vi "HighLVL.vi"() -> ()   [LabVIEW 2015]
uses:
  Public/Documents/SItoolkit/LabVIEW/Examples2015_6_0_2_9/Fast Examples/Open-Close Hardware/CamHandle.vi
  Public/Documents/SItoolkit/LabVIEW/Examples2015_6_0_2_9/Fast Examples/Cameras/NumericIndicator.vi
panel:
  out "Boolean":bool
  out "?":dbl
  out "Progress":u8(slide) scale=0.0..100.0
  out "Source Voltage":dbl
  out "Current (mA)":dbl
  out "Diode 2":string
  out "Diode 1":string
  out "Diode 3":string
  in  "File Path for Data Log":path=path "C:/Users/user/Dropbox (MIT)/stats/stats_00_00_00.txt"
  out "Source Mirror Position (mm)":dbl(slide) scale=0.0..50.0 scale format="%#.6g"
  out "Camera\nClosed":bool
  out "error out (Shutoff)":errorcluster
  out "Experiment Complete":bool
  out "Current File":string
  out "Logging Indicator":bool
  out "Current Set":dbl
  out "Current Frame":dbl
  in  "Anode":i32(knob) scale=1.0..6.0
  in  "Base FilePath (incrementing counter will be added to each following dataset)":path=path "C:/Users/Polarimetry/Desktop/High level experiment/exp"
  in  "Axis Positions":T1
  out "Experiment \nStarted":bool
  out "Estimated time (min)":dbl
  out "Initializing":bool
  out "error out (ADC)":errorcluster
  in  "begin":bool
  out "Read Temp":dbl(slide) scale=-50.0..20.0
  out "Camera open":bool
  out "Y Dimension":u32
  out "X Dimension":u32
  out "error out (Open Cam)":errorcluster
  in  "error in (no error)":errorcluster
  in  "Experiment Parameters":T2(tab)
  in  "Throwaway Frames":i32=1
  in  "# Frames":i32=10
  in  "ADC Speed (kHz)":i32=100
  in  "Exposure":i32=45
  in  "Cooling Temp":dbl=-50.0
  in  "Y2":i32=1300
  in  "Y1":i32=1
  in  "X2":i32=1340
  in  "X1":i32=1
  in  "x bin":u32=1
  in  "y bin":u32=1
  in  "min block":u32=2
  in  "Num Min Block":u32=5
  in  "ADC port":i32=1
  in  "ADC gain":i32=-1
  in  "Timing Mode":u32(ring)=1 items=["N/A", "Timed Mode/Free run", "Trigger First (only PM)", "Strobed/Ext Sync", "Bulb Mode (PM only)", "Variable Timed mode (PM only)", "Flash Mode (only some PM)"]
  in  "Motor Controls":T3(tab)
  in  "Detector Y#Steps":i32=1
  in  "Detector Y End":dbl
  in  "Detector Y Start":dbl
  in  "Detector X#Steps":i32=1
  in  "Detector X End":dbl
  in  "Detector X Start":dbl
  in  "Grating Angle#Steps":i32=1
  in  "Grating Angle End":dbl
  in  "Grating Angle Start":dbl
  in  "Grating Y#Steps":i32=1
  in  "Grating Y End":dbl
  in  "Grating Y Start":dbl
  in  "Grating X#Steps":i32=1
  in  "Grating X End":dbl
  in  "Grating X Start":dbl
  in  "Aperture X#Steps":i32=1
  in  "Aperture X End":dbl
  in  "Aperture X Start":dbl
  in  "Polarization #Steps":i32=1
  in  "Polarization End":dbl
  in  "Polarization Start":dbl
  in  "Mirror Angle #Steps":i32=1
  in  "Mirror Angle End":dbl
  in  "Mirror Angle Start":dbl
  in  "Mirror X #Steps":i32=1
  in  "Mirror X End":dbl
  in  "Mirror X Start":dbl
  # "These should be 1340 and 1300,\n if not, it is a demo cam"
  # "Note: Anode motor is not set up. \nOnly change this here if you manually changed the anode"
  # "Logging"
  # "ROI"
  # "Anode Control Not Supported.\nShut Off Voltage and Try Manually."
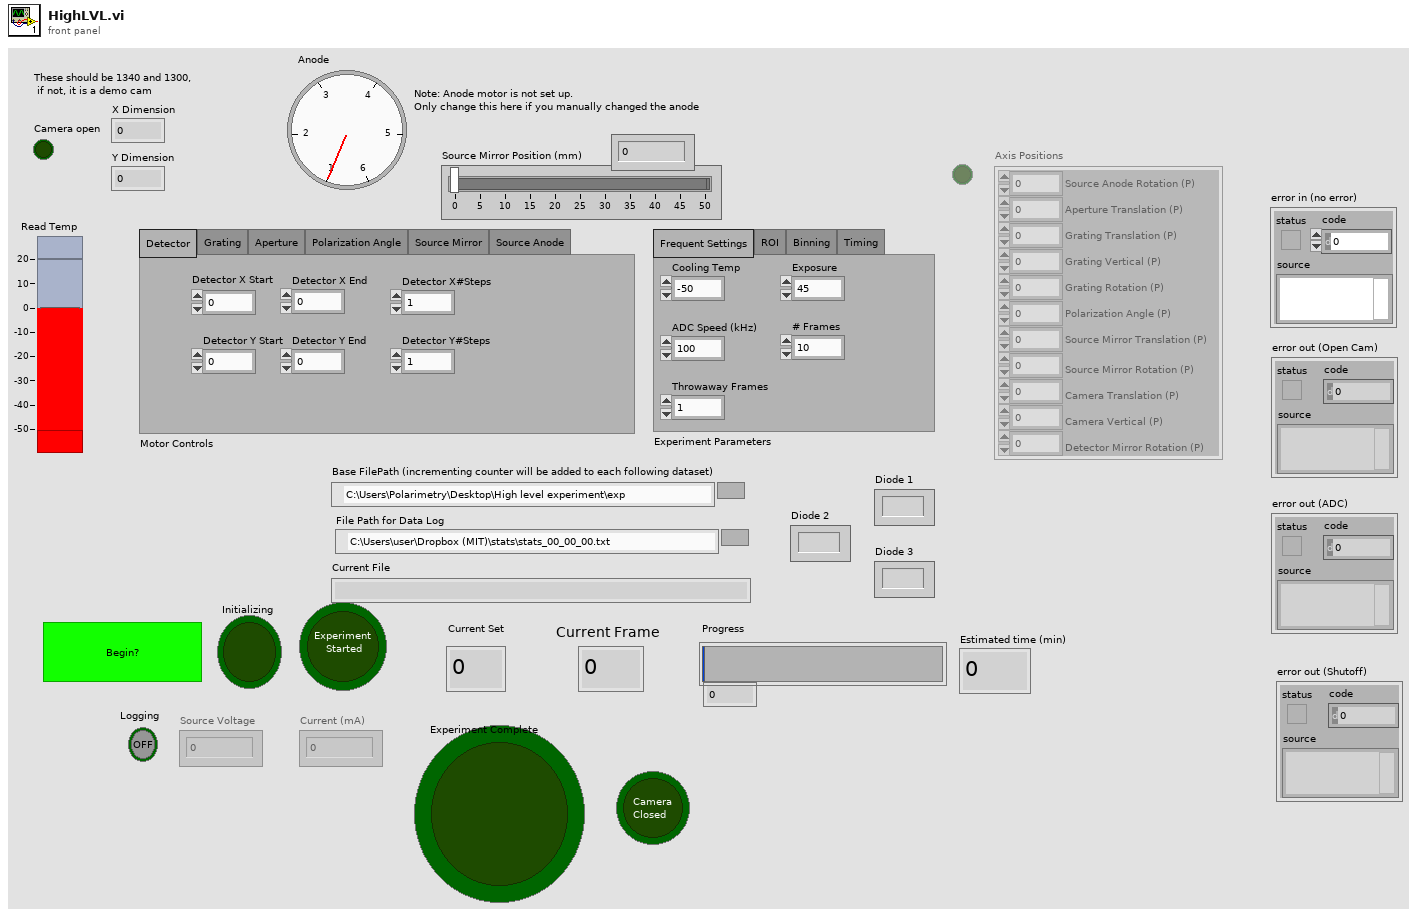
[diagram p1: front panel]
types:
  T1 = cluster{"Source Anode Rotation (P)":dbl, "Aperture Translation (P)":dbl, "Grating Translation (P)":dbl, "Grating Vertical (P)":dbl, "Grating Rotation (P)":dbl, "Polarization Angle (P)":dbl, "Source Mirror Translation (P)":dbl, "Source Mirror Rotation (P)":dbl, "Camera Translation (P)":dbl, "Camera Vertical (P) ":dbl, "Detector Mirror Rotation (P)":dbl}
  T2 = enum32{"Frequent Settings", "ROI", "Binning", "Timing"}
  T3 = enum32{"Detector", "Grating", "Aperture", "Polarization Angle", "Source Mirror", "Source Anode"}
  T4 = cluster{"Axis Prefix":string, bool, i32, i32, i32, i32}
  T5 = cluster{"Axis Prefix":string, bool, i32, i32, i32, dbl}
  T6 = cluster{"Axis Prefix":string, bool, i32, dbl, i32, i32}
  T7 = enum16{"open", "replace", "create", "open or create", "replace or create", "replace or create with confirmation"}
  T8 = cluster{"Detector X Start":dbl, "Detector Y Start":dbl, "Grating X Start":dbl, "Grating Y Start":dbl, "Grating Angle Start":dbl, "Aperture X Start":dbl, "Polarization Start":dbl, "Mirror X Start":dbl, "Mirror Angle Start":dbl}
  T9 = cluster{"Detector X End":dbl, "Detector Y End":dbl, "Grating X End":dbl, "Grating Y End":dbl, "Grating Angle End":dbl, "Aperture X End":dbl, "Polarization End":dbl, "Mirror X End":dbl, "Mirror Angle End":dbl}
  T10 = cluster{"Detector X#Steps":i32, "Detector Y#Steps":i32, "Grating X#Steps":i32, "Grating Y#Steps":i32, "Grating Angle#Steps":i32, "Aperture X#Steps":i32, "Polarization #Steps":i32, "Mirror X #Steps":i32, "Mirror Angle #Steps":i32}
  T11 = cluster{"ADC Speed (kHz)":i32, "Throwaway Frames":i32, "# Frames":i32, "Exposure":i32, "Cooling Temp":dbl}
  T12 = cluster{"X1":i32, "X2":i32, "x bin":u32, "Y1":i32, "Y2":i32, "y bin":u32}
  T13 = cluster{"Increment":dbl, "Increment":dbl, "Increment":dbl, "Increment":dbl, "Increment":dbl, "Increment":dbl, "Increment":dbl, "Increment":dbl, "Increment":dbl}
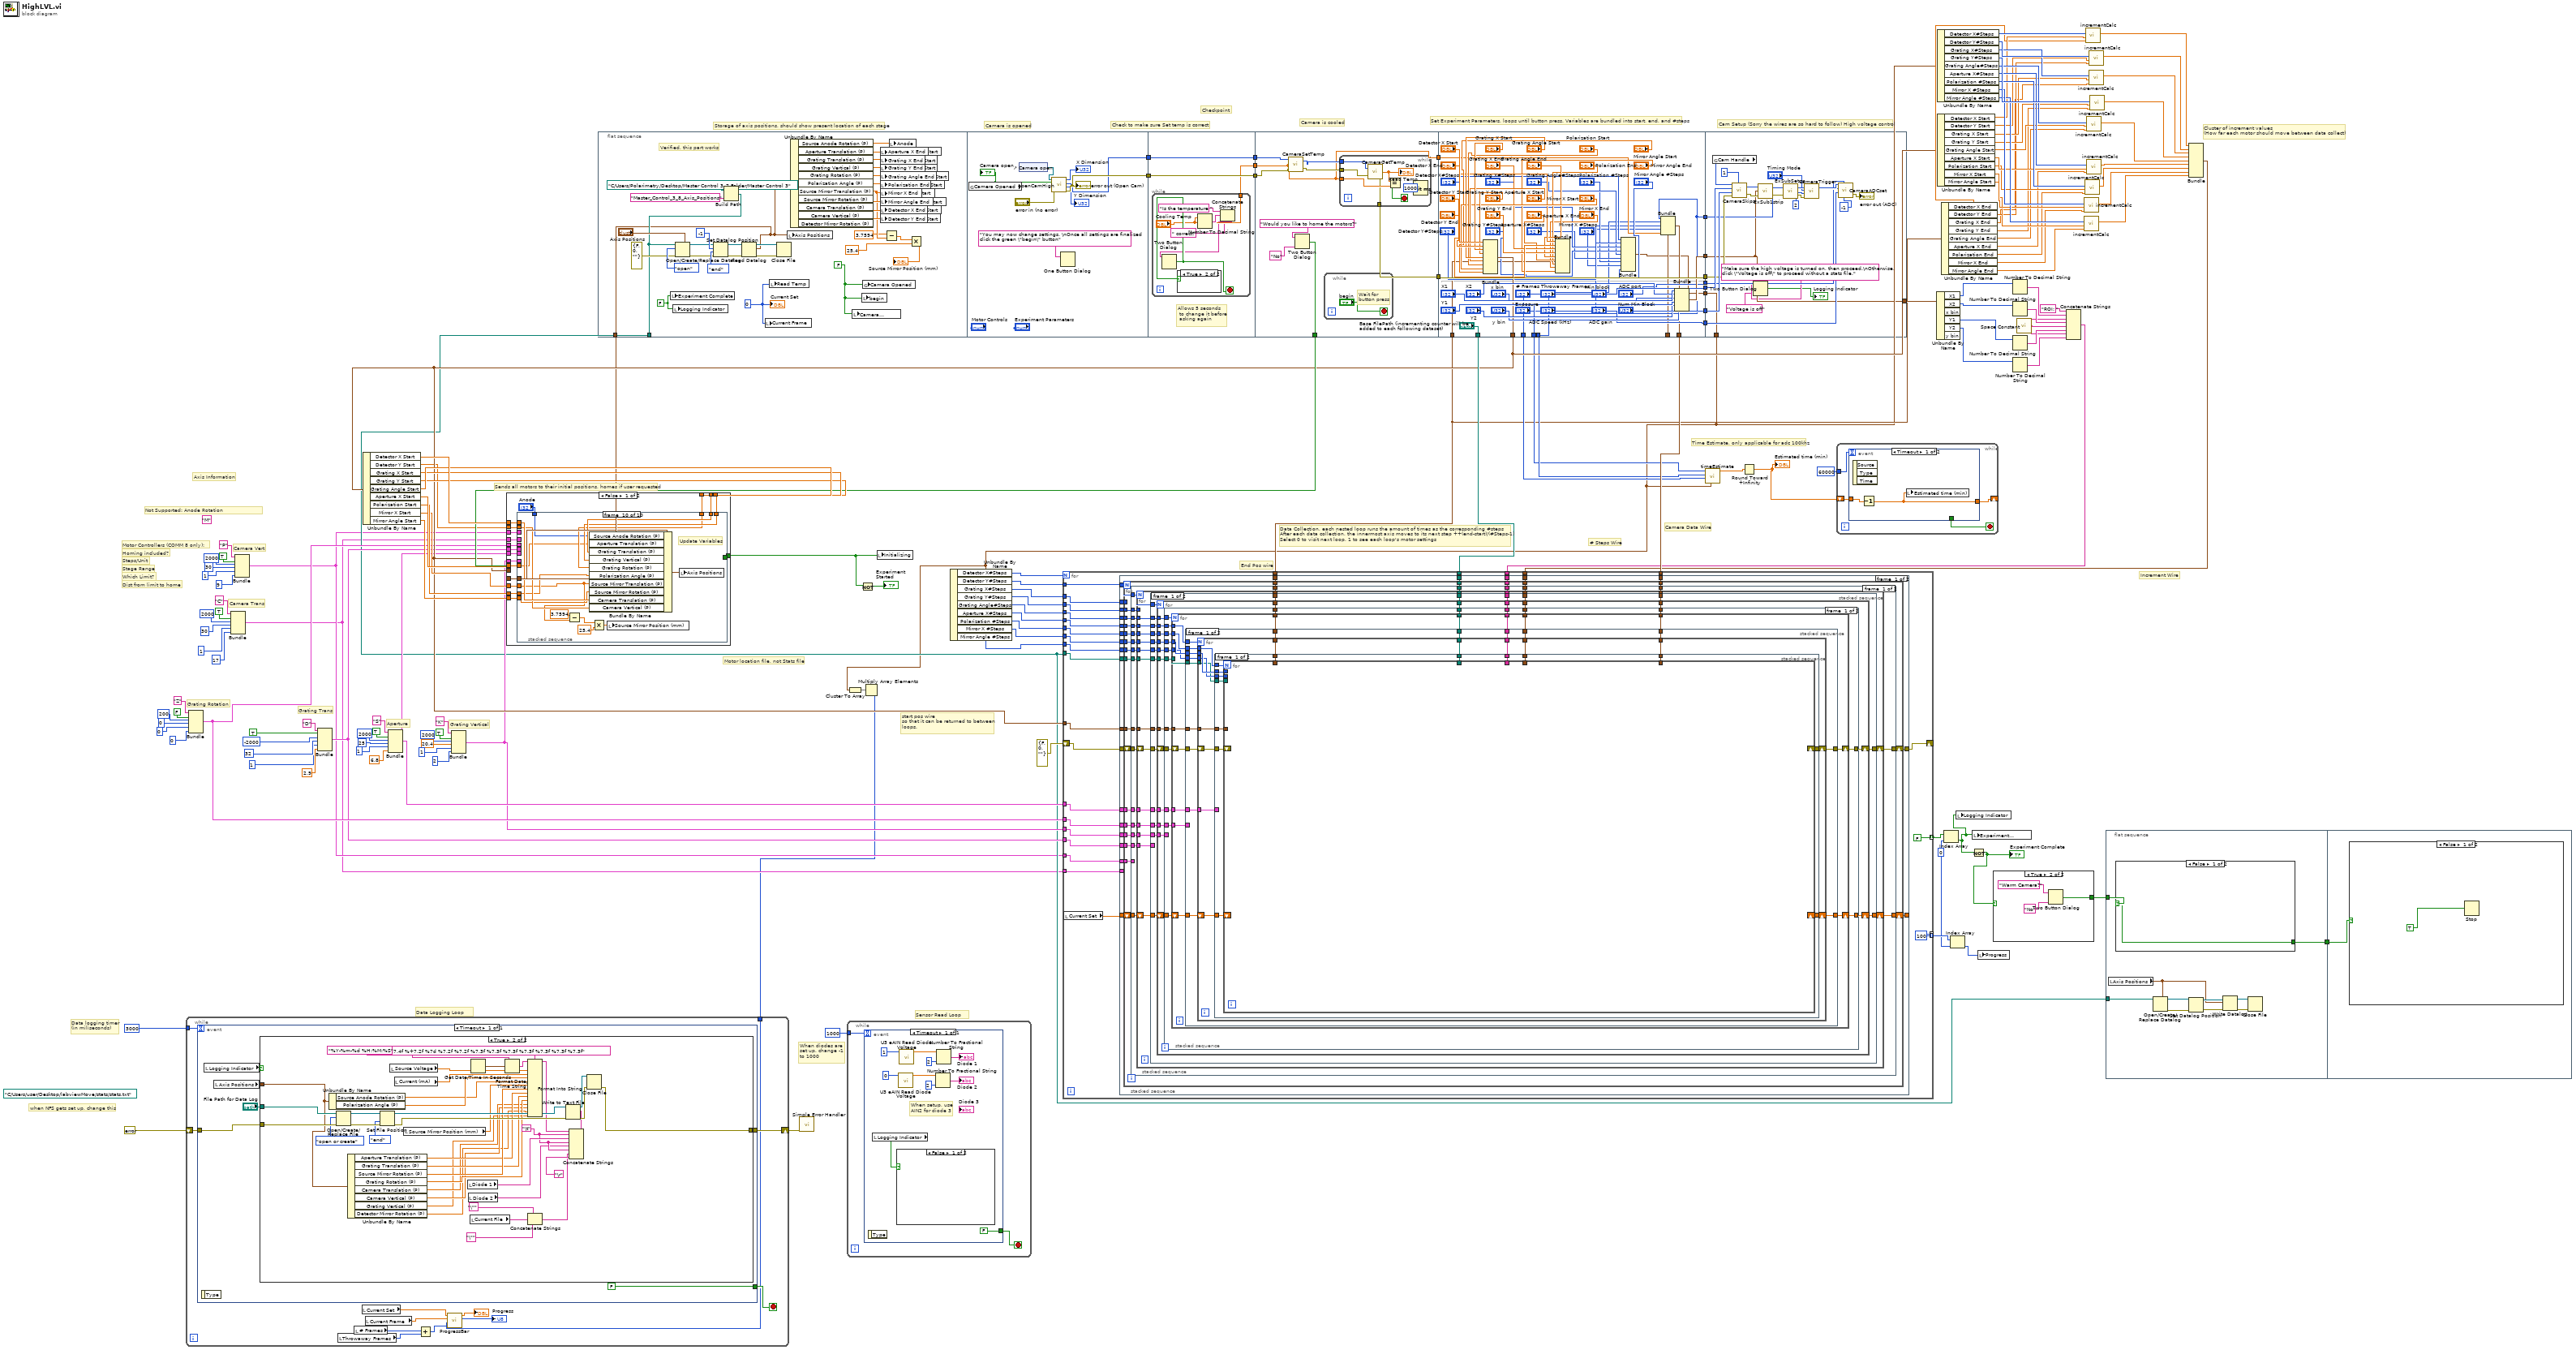
[diagram p0: block diagram]
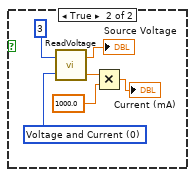
[diagram p2: hidden frame]
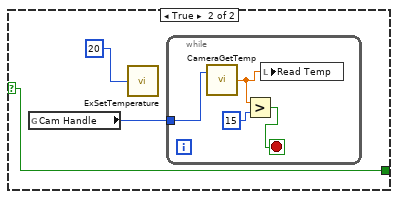
[diagram p4: hidden frame]
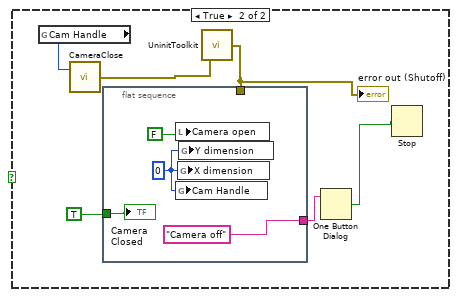
[diagram p5: hidden frame]
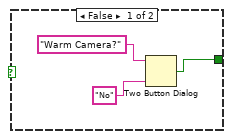
[diagram p6: hidden frame]
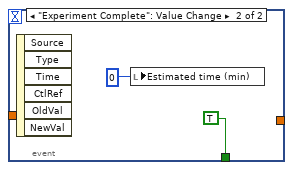
[diagram p7: hidden frame]
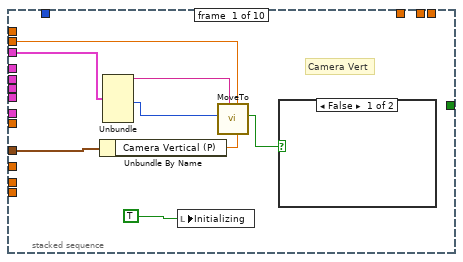
[diagram p8: hidden frame]
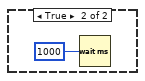
[diagram p9: hidden frame]
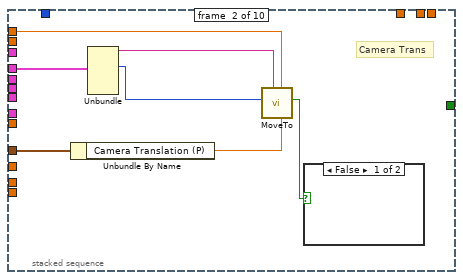
[diagram p10: hidden frame]
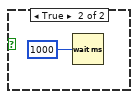
[diagram p11: hidden frame]
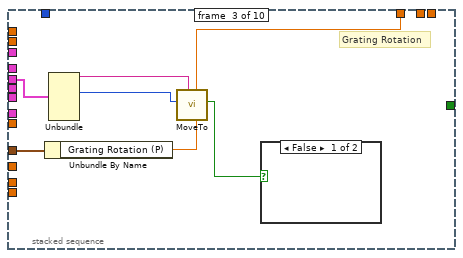
[diagram p12: hidden frame]
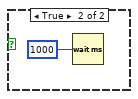
[diagram p13: hidden frame]
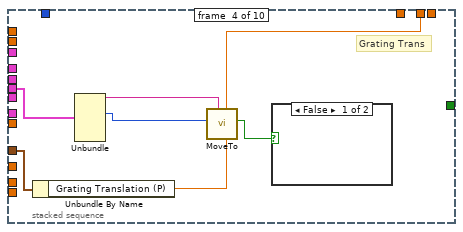
[diagram p14: hidden frame]
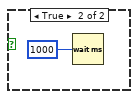
[diagram p15: hidden frame]
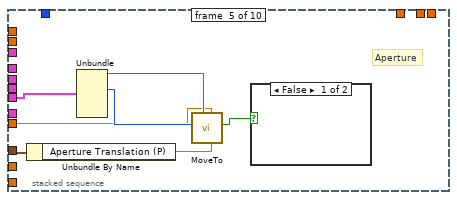
[diagram p16: hidden frame]
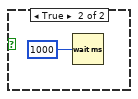
[diagram p17: hidden frame]
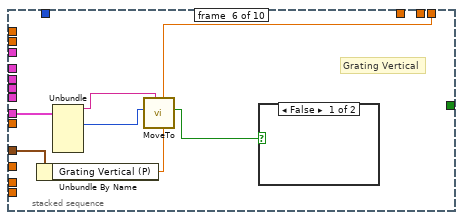
[diagram p18: hidden frame]
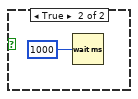
[diagram p19: hidden frame]
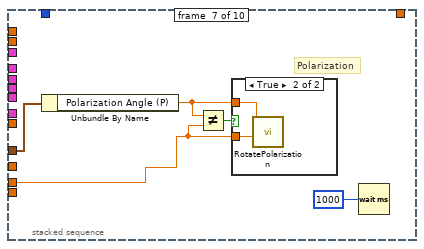
[diagram p20: hidden frame]
diagram:
  (unwired) path "C:/Users/user/Desktop/labviewMove/stats/stats.txt" ("file path (use dialog)")
  w3 = 0
  (unwired) "M" ("Axis Prefix")
  # "when NFS gets set up, change this"
  # "When diodes are \nset up, change -1 \nto 1000"
  # "Sensor Read Loop"
  # "Data Logging Loop"
  # "Data logging timer\n(in miliseconds)"
  # "Checkpoint"
  # "Motor location file, not Stats file"
  # "Increment Wire"
  # "Camera Data Wire"
  # "# Steps Wire"
  # "End Pos wire"
  # "start pos wire\nso that it can be returned to between\nloops."
  # "Cluster of increment values \n(How far each motor should move between data collect)"
  # "Storage of axis positions, should show present location of each stage"
  # "Data Collection, each nested loop runs the amount of times as the corresponding #steps\nAfter each data collection, the innermost axis moves to its next step ++(end-start)/(#Steps-1)\nSelect 0 to visit next loop, 1 to see each loop's motor settings"
  # "Time Estimate, only applicable for adc 100khz"
  # "Axis Information"
  # "Camera Vert"
  # "Camera Trans"
  # "Grating Rotation"
  # "Grating Vertical"
  # "Grating Trans"
  # "Aperture"
  # "Dist from limit to home"
  # "Not Supported: Anode Rotation"
  # "Which Limit?"
  # "Stage Range"
  # "Steps/Unit"
  # "Homing included?"
  # "Motor Controllers (COMM 8 only):"
  # "Sends all motors to their initial positions, homes if user requested"
  # "Cam Setup (Sorry the wires are so hard to follow) High voltage control"
  # "Check to make sure Set temp is correct"
  # "Set Experiment Parameters, loops until button press. Variables are bundled into start, end, and #steps"
  # "Camera is cooled"
  # "Camera is opened"
  n1 = Bundle("Axis Prefix"="Z", FALSE, 200, 0, 0, 0) -> (w29:T4)  [unwired: 1 in]
  n2 = Bundle("Axis Prefix"="C", TRUE, 2000, 30, 1, 17) -> (w11:T4)  [unwired: 1 in]
  n3 = Bundle("Axis Prefix"="P", TRUE, 2000, 30, 1, 9) -> (w12:T4)  [unwired: 1 in]
  n4 = Bundle("Axis Prefix"="D", TRUE, -2000, 32, 1, 2.9) -> (w22:T5)  [unwired: 1 in]
  n5 = Unbundle By Name(w50) -> ("Detector X Start"=w145:dbl, "Detector Y Start"=w23:dbl, "Grating X Start"=w107:dbl, "Grating Y Start"=w105:dbl, "Grating Angle Start"=w108:dbl, "Aperture X Start"=w106:dbl, "Polarization Start"=w90:dbl, "Mirror X Start"=w89:dbl, "Mirror Angle Start"=w88:dbl)
  n6 = Bundle("Axis Prefix"="S", TRUE, 2000, 25, 1, 6.8) -> (w30:T5)  [unwired: 1 in]
  n7 = Bundle("Axis Prefix"="K", TRUE, 2000, 20.4, 1, 2) -> (w28:T6)  [unwired: 1 in]
  n8 = case shown="False" w51 {
    tunnel: w145 -> [w173 w279]
    tunnel: w12 -> [w172 w278]
    tunnel: w11 -> [w168 w277]
    tunnel: w29 -> [w169 w276]
    tunnel: w22 -> [w166 w275]
    tunnel: w30 -> [w164 w274]
    tunnel: w28 -> [w162 w273]
    tunnel: w23 -> [w170 w272]
    tunnel: w108 -> [w167 w271]
    tunnel: w107 -> [w165 w270]
    tunnel: w106 -> [w163 w269]
    tunnel: w105 -> [w161 w268]
    tunnel: [w157 w267] -> w95
    tunnel: w21 -> [w171 w266]
    tunnel: w90 -> [w159 w265]
    tunnel: w89 -> [w160 w264]
    tunnel: w88 -> [w158 w263]
    tunnel: w50 -> [_ w262]
    frame False {
      n9 = stacked-sequence {
        tunnel: w173 -> [_ w183 _ _ _ _ _ _ _ w259]
        tunnel: w172 -> [w181 _ _ _ _ _ _ _ _ _]
        tunnel: w171 -> [w178 w187 w195 w201 w213 w218 w227 w233 w241 w260]
        tunnel: w170 -> [w174 _ _ _ _ _ _ _ _ w258]
        tunnel: w169 -> [_ _ w191 _ _ _ _ _ _ _]
        tunnel: w168 -> [_ w185 _ _ _ _ _ _ _ _]
        tunnel: w167 -> [_ _ w193 _ _ _ _ _ _ w255]
        tunnel: w166 -> [_ _ _ w205 _ _ _ _ _ _]
        tunnel: w165 -> [_ _ _ w202 _ _ _ _ _ w257]
        tunnel: w164 -> [_ _ _ _ w211 _ _ _ _ _]
        tunnel: w163 -> [_ _ _ _ w207 _ _ _ _ w253]
        tunnel: w162 -> [_ _ _ _ _ w221 _ _ _ _]
        tunnel: w161 -> [_ _ _ _ _ w216 _ _ _ w256]
        tunnel: "Anode" -> [_ _ _ _ _ _ _ _ _ w254]
        tunnel: w160 -> [_ _ _ _ _ _ _ w231 _ w246]
        tunnel: w159 -> [_ _ _ _ _ _ w224 _ _ w252]
        tunnel: w158 -> [_ _ _ _ _ _ _ _ w237 w251]
        tunnel: [_ _ _ _ _ _ _ _ FALSE _] -> w157
        frame #0 {
          # "Camera Vert"
          n10 = Unbundle By Name(w178) -> ("Camera Vertical (P)"=w177:dbl)
          n11 = Unbundle(w181) -> ("Axis Prefix"=w180:string, w179:i32)  [unwired: 4 out]
          n12 = local write "Initializing"(TRUE) -> ()
          n13 = call "MoveTo.vi"("Curr Pos"=w177, "Desired Pos"=w174, "Axis Name"=w180, "Steps/unit"=w179) -> ("Anything move?"=w176:bool)  [unwired: 7 in]
          n14 = case shown="False" w176 {
            frame False {
            }
            frame True {
              n15 = Wait (ms)(milliseconds to wait=1000) -> ()  [unwired: 1 out]
            }
          }
        }
        frame #1 {
          # "Camera Trans"
          n16 = Unbundle By Name(w187) -> ("Camera Translation (P)"=w186:dbl)
          n17 = Unbundle(w185) -> ("Axis Prefix"=w189:string, w188:i32)  [unwired: 4 out]
          n18 = call "MoveTo.vi"("Curr Pos"=w186, "Desired Pos"=w183, "Axis Name"=w189, "Steps/unit"=w188) -> ("Anything move?"=w184:bool)  [unwired: 7 in]
          n19 = case shown="False" w184 {
            frame False {
            }
            frame True {
              n20 = Wait (ms)(milliseconds to wait=1000) -> ()  [unwired: 1 out]
            }
          }
        }
        frame #2 {
          # "Grating Rotation"
          n21 = Unbundle By Name(w195) -> ("Grating Rotation (P)"=w194:dbl)
          n22 = Unbundle(w191) -> ("Axis Prefix"=w197:string, w196:i32)  [unwired: 4 out]
          n23 = call "MoveTo.vi"("Curr Pos"=w194, "Desired Pos"=w193, "Axis Name"=w197, "Steps/unit"=w196) -> ("Anything move?"=w192:bool)  [unwired: 7 in]
          n24 = case shown="False" w192 {
            frame False {
            }
            frame True {
              n25 = Wait (ms)(milliseconds to wait=1000) -> ()  [unwired: 1 out]
            }
          }
        }
        frame #3 {
          # "Grating Trans"
          n26 = Unbundle By Name(w201) -> ("Grating Translation (P)"=w200:dbl)
          n27 = Unbundle(w205) -> ("Axis Prefix"=w204:string, w203:i32)  [unwired: 4 out]
          n28 = call "MoveTo.vi"("Curr Pos"=w200, "Desired Pos"=w202, "Axis Name"=w204, "Steps/unit"=w203) -> ("Anything move?"=w199:bool)  [unwired: 7 in]
          n29 = case shown="False" w199 {
            frame False {
            }
            frame True {
              n30 = Wait (ms)(milliseconds to wait=1000) -> ()  [unwired: 1 out]
            }
          }
        }
        frame #4 {
          # "Aperture"
          n31 = Unbundle By Name(w213) -> ("Aperture Translation (P)"=w212:dbl)
          n32 = Unbundle(w211) -> ("Axis Prefix"=w210:string, w209:i32)  [unwired: 4 out]
          n33 = call "MoveTo.vi"("Curr Pos"=w212, "Desired Pos"=w207, "Axis Name"=w210, "Steps/unit"=w209) -> ("Anything move?"=w208:bool)  [unwired: 7 in]
          n34 = case shown="False" w208 {
            frame False {
            }
            frame True {
              n35 = Wait (ms)(milliseconds to wait=1000) -> ()  [unwired: 1 out]
            }
          }
        }
        frame #5 {
          # "Grating Vertical"
          n36 = Unbundle By Name(w218) -> ("Grating Vertical (P)"=w217:dbl)
          n37 = Unbundle(w221) -> ("Axis Prefix"=w220:string, w219:i32)  [unwired: 4 out]
          n38 = call "MoveTo.vi"("Curr Pos"=w217, "Desired Pos"=w216, "Axis Name"=w220, "Steps/unit"=w219) -> ("Anything move?"=w215:bool)  [unwired: 7 in]
          n39 = case shown="False" w215 {
            frame False {
            }
            frame True {
              n40 = Wait (ms)(milliseconds to wait=1000) -> ()  [unwired: 1 out]
            }
          }
        }
        frame #6 {
          # "Polarization"
          n41 = Unbundle By Name(w227) -> ("Polarization Angle (P)"=w225:dbl)
          n42 = Not Equal?(x=w225, y=w224) -> (x != y?=w223:bool)
          n43 = case shown="True" w223 {
            tunnel: w224 -> [_ w229]
            tunnel: w225 -> [_ w228]
            frame False {
            }
            frame True {
              n44 = call "RotatePolarization.vi"("End Pos"=w229, "curr pos"=w228) -> ()  [unwired: 9 in, 1 out]
            }
          }
          n45 = Wait (ms)(milliseconds to wait=1000) -> ()  [unwired: 1 out]
        }
        frame #7 {
          # "Mirror X"
          n46 = Unbundle By Name(w233) -> ("Source Mirror Translation (P)"=w230:dbl)
          n47 = Not Equal?(x=w230, y=w231) -> (x != y?=w232:bool)
          n48 = case shown="False" w232 {
            tunnel: w231 -> [_ w236]
            tunnel: w230 -> [_ w235]
            frame False {
            }
            frame True {
              n49 = call "SourceMirrorTrans.vi"("EndPos"=w236, "CurrPos"=w235) -> ()  [unwired: 9 in, 1 out]
            }
          }
          n50 = Wait (ms)(milliseconds to wait=5000) -> ()  [unwired: 1 out]
        }
        frame #8 {
          # "Mirror Angle"
          n51 = Unbundle By Name(w241) -> ("Source Mirror Rotation (P)"=w238:dbl)
          n52 = Not Equal?(x=w238, y=w237) -> (x != y?=w239:bool)
          n53 = case shown="False" w239 {
            tunnel: w238 -> [_ w244]
            tunnel: w237 -> [_ w243]
            frame False {
            }
            frame True {
              n54 = call "SourceMirrorAngle.vi"("EndPos"=w243, "CurrPos"=w244) -> ()  [unwired: 9 in, 1 out]
            }
          }
          n55 = Wait (ms)(milliseconds to wait=1000) -> ()  [unwired: 1 out]
        }
        frame #9 {
          # "Update Variables"
          n56 = Subtract(x=3.7594, y=w246) -> (x-y=w245:dbl)
          n57 = Bundle By Name(cluster=w260, "Source Anode Rotation (P)"=w254, "Aperture Translation (P)"=w253, "Grating Translation (P)"=w257, "Grating Vertical (P)"=w256, "Grating Rotation (P)"=w255, "Polarization Angle (P)"=w252, "Source Mirror Translation (P)"=w246, "Source Mirror Rotation (P)"=w251, "Camera Translation (P)"=w259, "Camera Vertical (P)"=w258) -> (w250:T1)
          n58 = Multiply(x=w245, y=25.4) -> (x*y=w248:dbl)
          n59 = local write "Source Mirror Position (mm)"(w248) -> ()
          n60 = local write "Axis Positions"(w250) -> ()
        }
      }
    }
    frame True {
      n61 = local read "Anode"() -> (w261:i32)
      n62 = stacked-sequence {
        tunnel: w279 -> [_ w290 _ _ _ _ _ _ _ w367]
        tunnel: w278 -> [w280 _ _ _ _ _ _ _ _ _]
        tunnel: w277 -> [_ w291 _ _ _ _ _ _ _ _]
        tunnel: w276 -> [_ _ w302 _ _ _ _ _ _ _]
        tunnel: w275 -> [_ _ _ w311 _ _ _ _ _ _]
        tunnel: w274 -> [_ _ _ _ w320 _ _ _ _ _]
        tunnel: w273 -> [_ _ _ _ _ w329 _ _ _ _]
        tunnel: w272 -> [w283 _ _ _ _ _ _ _ _ w366]
        tunnel: w271 -> [_ _ w301 _ _ _ _ _ _ w363]
        tunnel: w270 -> [_ _ _ w310 _ _ _ _ _ w365]
        tunnel: w269 -> [_ _ _ _ w319 _ _ _ _ w362]
        tunnel: w268 -> [_ _ _ _ _ w328 _ _ _ w364]
        tunnel: [_ _ _ _ _ _ _ _ FALSE _] -> w267
        tunnel: w266 -> [_ _ w299 _ _ _ w339 w344 w349 w368]
        tunnel: w262 -> [_ _ _ _ _ _ _ _ _ _]
        tunnel: w265 -> [_ _ _ _ _ _ w338 _ _ w360]
        tunnel: w264 -> [_ _ _ _ _ _ _ w343 _ w353]
        tunnel: w263 -> [_ _ _ _ _ _ _ _ w348 w361]
        tunnel: w261 -> [_ _ _ _ _ _ _ _ _ w359]
        frame #0 {
          # "Camera Vert"
          n63 = Unbundle(w280) -> ("Axis Prefix"=w288:string, w281:bool, w287:i32, w286:i32, w285:i32, w284:i32)
          "Initializing" <- w281
          n64 = call "HomeMoveTo.vi"("Start Pos"=w283, "Distance from lim to home"=w284, "Axis Name"=w288, "Which Limit"=w285, "Stage Range"=w286, "Steps/unit"=w287, "Homes?"=w281) -> ()  [unwired: 5 in]
          n65 = Wait (ms)(milliseconds to wait=1000) -> ()  [unwired: 1 out]
        }
        frame #1 {
          # "Camera Trans"
          n66 = Unbundle(w291) -> ("Axis Prefix"=w297:string, w296:bool, w295:i32, w294:i32, w293:i32, w292:i32)
          n67 = call "HomeMoveTo.vi"("Start Pos"=w290, "Distance from lim to home"=w292, "Axis Name"=w297, "Which Limit"=w293, "Stage Range"=w294, "Steps/unit"=w295, "Homes?"=w296) -> ()  [unwired: 5 in]
          n68 = Wait (ms)(milliseconds to wait=1000) -> ()  [unwired: 1 out]
        }
        frame #2 {
          # "Grating Rotation"
          n69 = Unbundle By Name(w299) -> ("Grating Rotation (P)"=w298:dbl)
          n70 = Unbundle(w302) -> ("Axis Prefix"=w308:string, w307:bool, w306:i32, w305:i32, w304:i32, w303:i32)
          n71 = call "HomeMoveTo.vi"("Curr Pos"=w298, "Start Pos"=w301, "Distance from lim to home"=w303, "Axis Name"=w308, "Which Limit"=w304, "Stage Range"=w305, "Steps/unit"=w306, "Homes?"=w307) -> ()  [unwired: 4 in]
          n72 = Wait (ms)(milliseconds to wait=1000) -> ()  [unwired: 1 out]
        }
        frame #3 {
          # "Grating Translation"
          n73 = Unbundle(w311) -> ("Axis Prefix"=w317:string, w316:bool, w315:i32, w314:i32, w313:i32, w312:dbl)
          n74 = call "HomeMoveTo.vi"("Start Pos"=w310, "Distance from lim to home"=w312, "Axis Name"=w317, "Which Limit"=w313, "Stage Range"=w314, "Steps/unit"=w315, "Homes?"=w316) -> ()  [unwired: 5 in]
          n75 = Wait (ms)(milliseconds to wait=1000) -> ()  [unwired: 1 out]
        }
        frame #4 {
          # "Aperture Translation"
          n76 = Unbundle(w320) -> ("Axis Prefix"=w326:string, w325:bool, w324:i32, w323:i32, w322:i32, w321:dbl)
          n77 = call "HomeMoveTo.vi"("Start Pos"=w319, "Distance from lim to home"=w321, "Axis Name"=w326, "Which Limit"=w322, "Stage Range"=w323, "Steps/unit"=w324, "Homes?"=w325) -> ()  [unwired: 5 in]
          n78 = Wait (ms)(milliseconds to wait=1000) -> ()  [unwired: 1 out]
        }
        frame #5 {
          # "Grating Vertical"
          n79 = Unbundle(w329) -> ("Axis Prefix"=w335:string, w334:bool, w333:i32, w332:dbl, w331:i32, w330:i32)
          n80 = call "HomeMoveTo.vi"("Start Pos"=w328, "Distance from lim to home"=w330, "Axis Name"=w335, "Which Limit"=w331, "Stage Range"=w332, "Steps/unit"=w333, "Homes?"=w334) -> ()  [unwired: 5 in]
          n81 = Wait (ms)(milliseconds to wait=1000) -> ()  [unwired: 1 out]
        }
        frame #6 {
          (unwired) 5
          # "Start-cur"
          # "Test this, it could move \nit before it is told how far"
          # "Polarization"
          n82 = Unbundle By Name(w339) -> ("Polarization Angle (P)"=w336:dbl)
          n83 = Subtract(x=w338, y=w336) -> (x-y=w337:dbl)
          n84 = call "RotatePolarization.vi"("End Pos"=w337, "curr pos"=w336) -> ()  [unwired: 9 in, 1 out]
          n85 = Wait (ms)(milliseconds to wait=1000) -> ()  [unwired: 1 out]
        }
        frame #7 {
          # "Start-cur"
          # "Test this, it could move \nit before it is told how far"
          # "Mirror X"
          n86 = Unbundle By Name(w344) -> ("Source Mirror Translation (P)"=w342:dbl)
          n87 = Subtract(x=w343, y=w342) -> (x-y=w341:dbl)
          n88 = call "SourceMirrorTrans.vi"("EndPos"=w341, "CurrPos"=w342) -> ()  [unwired: 9 in, 1 out]
          n89 = Wait (ms)(milliseconds to wait=1000) -> ()  [unwired: 1 out]
        }
        frame #8 {
          # "Start-cur"
          # "Test this, it could move \nit before it is told how far"
          # "Mirror Angle"
          n90 = Unbundle By Name(w349) -> ("Source Mirror Rotation (P)"=w347:dbl)
          n91 = Subtract(x=w348, y=w347) -> (x-y=w346:dbl)
          n92 = call "SourceMirrorAngle.vi"("EndPos"=w346, "CurrPos"=w347) -> ()  [unwired: 9 in, 1 out]
          n93 = Wait (ms)(milliseconds to wait=1000) -> ()  [unwired: 1 out]
        }
        frame #9 {
          n94 = Bundle By Name(cluster=w368, "Source Anode Rotation (P)"=w359, "Aperture Translation (P)"=w362, "Grating Translation (P)"=w365, "Grating Vertical (P)"=w364, "Grating Rotation (P)"=w363, "Polarization Angle (P)"=w360, "Source Mirror Translation (P)"=w353, "Source Mirror Rotation (P)"=w361, "Camera Translation (P)"=w367, "Camera Vertical (P)"=w366) -> (w358:T1)
          n95 = local write "Axis Positions"(w358) -> ()
          n96 = Subtract(x=3.7594, y=w353) -> (x-y=w352:dbl)
          n97 = Wait (ms)(milliseconds to wait=10000) -> ()  [unwired: 1 out]
          n98 = Multiply(x=25.4, y=w352) -> (x*y=w356:dbl)
          n99 = local write "Source Mirror Position (mm)"(w356) -> ()
        }
      }
    }
  }
  n100 = flat-sequence {
    tunnel: [w387] -> w17
    tunnel: [w378] -> w21
    tunnel: [w405] -> w155
    tunnel: [w401] -> w7
    tunnel: w155 -> [w411]
    tunnel: [w411] -> w154
    tunnel: [w410] -> w27
    tunnel: [w409] -> w8
    tunnel: w7 -> [w409]
    tunnel: w154 -> [w421]
    tunnel: [w427] -> w151
    tunnel: [w424] -> w51
    tunnel: [w419] -> w38
    tunnel: w27 -> [w419]
    tunnel: w8 -> [w423]
    tunnel: ["min block"] -> w153
    tunnel: ["Num Min Block"] -> w152
    tunnel: w151 -> [w482]
    tunnel: [w482] -> w150
    tunnel: [w475] -> w149
    tunnel: ["ADC gain"] -> w148
    tunnel: ["ADC Speed (kHz)"] -> w147
    tunnel: ["ADC port"] -> w146
    tunnel: [w463] -> w50
    tunnel: ["Base FilePath (incrementing counter will be added to each following dataset)"] -> w91
    tunnel: [w443] -> w31
    tunnel: w38 -> [w441]
    tunnel: [w440] -> _
    tunnel: [w440] -> w37
    tunnel: ["Throwaway Frames"] -> w35
    tunnel: ["# Frames"] -> w34
    tunnel: ["Exposure"] -> w33
    tunnel: [w436] -> w6
    tunnel: w153 -> [w507]
    tunnel: w152 -> [w506]
    tunnel: w150 -> [w504]
    tunnel: w149 -> [w489]
    tunnel: w148 -> [w490]
    tunnel: w147 -> [w494]
    tunnel: w146 -> [w492]
    tunnel: [w489] -> w43
    tunnel: w6 -> [w485]
    tunnel: [w485] -> w5
    frame #0 {
      w373 = FALSE
      w374 = FALSE
      w372 = 0
      # "Verified, this part works"
      n101 = local write "Experiment Complete"(w374) -> ()
      n102 = local write "Logging Indicator"(w374) -> ()
      n103 = Build Path(base path=path "C:/Users/Polarimetry/Desktop/Master Control 3_7 Folder/Master Control 3", name or relative path="Master_Control_3_8_Axis_Positions") -> (appended path=w387:path)
      n104 = Open/Create/Replace Datalog(5:"Axis Positions", 8:errorcluster {"status"=FALSE, "code"=0, "source"=""} ("error constant"), 10:T7."open" ("operation (0:open)"), 11:w387) -> (0:w392:errorcluster, 3:w393:refnum<k1>)  [unwired: 2 in, 1 out]
      n105 = Set Datalog Position(4:w392, 5:enum16{"start", "end", "current"}."end" ("from (0:start)"), 6:i64 -1 ("offset (in records) (0)"), 7:w393) -> (0:w391:errorcluster, 3:w397:refnum<k1>)
      n106 = Read Datalog(4:w391, 7:w397) -> (0:w390:errorcluster, 2:w378:T1, 3:w398:refnum<k1>)  [unwired: 1 in]
      n107 = local write "Current Frame"(w372) -> ()
      n108 = local write "Read Temp"(w372) -> ()
      n109 = Close File(refnum=w398, error in=w390) -> ()  [unwired: 2 out]
      n110 = local write "Axis Positions"(w378) -> ()
      n111 = Unbundle By Name(w378) -> ("Source Anode Rotation (P)"=w377:dbl, "Aperture Translation (P)"=w381:dbl, "Grating Translation (P)"=w384:dbl, "Grating Vertical (P)"=w383:dbl, "Grating Rotation (P)"=w382:dbl, "Polarization Angle (P)"=w380:dbl, "Source Mirror Translation (P)"=w370:dbl, "Source Mirror Rotation (P)"=w379:dbl, "Camera Translation (P)"=w386:dbl, "Camera Vertical (P)"=w385:dbl)  [unwired: 1 out]
      n112 = local write "Camera\nClosed"(w373) -> ()
      n113 = local write "begin"(w373) -> ()
      n114 = global write "CamHandle.vi" "Camera Opened"(w373) -> ()
      n115 = local write "Aperture X End"(w381) -> ()
      n116 = local write "Grating X End"(w384) -> ()
      n117 = local write "Grating Y End"(w383) -> ()
      n118 = local write "Grating Angle End"(w382) -> ()
      n119 = local write "Polarization End"(w380) -> ()
      n120 = local write "Mirror X End"(w370) -> ()
      n121 = local write "Mirror Angle End"(w379) -> ()
      n122 = local write "Detector X End"(w386) -> ()
      n123 = local write "Detector Y End"(w385) -> ()
      n124 = Subtract(x=3.7594, y=w370) -> (x-y=w371:dbl)
      n125 = local write "Anode"(w377) -> ()
      n126 = local write "Aperture X Start"(w381) -> ()
      n127 = local write "Grating X Start"(w384) -> ()
      n128 = local write "Grating Y Start"(w383) -> ()
      n129 = local write "Grating Angle Start"(w382) -> ()
      n130 = local write "Mirror X Start"(w370) -> ()
      n131 = local write "Detector Y Start"(w385) -> ()
      n132 = local write "Polarization Start"(w380) -> ()
      n133 = local write "Mirror Angle Start"(w379) -> ()
      n134 = local write "Detector X Start"(w386) -> ()
      n135 = Multiply(x=w371, y=25.4) -> (x*y=→"Source Mirror Position (mm)":dbl)
      "Current Set" <- w372
    }
    frame #1 {
      n136 = global read "CamHandle.vi" "Camera Opened"() -> (w408:bool)
      "Camera open" <- w408
      n137 = control-ref of="Camera open"() -> (w407:refnum<vi>)
      n138 = call "openCamHigh.vi"("error in (no error)"="error in (no error)", "Camera Opened"=w408, "Boolean in"=w407) -> ("error out"=w405:errorcluster, "Cam Handle"=w401:u32, "Ydim"=→"Y Dimension":u32, "Xdim"=→"X Dimension":u32)  [unwired: 5 in]
      "error out (Open Cam)" <- w405
      n139 = One Button Dialog(message="You may now change settings. \nOnce all settings are finalized click the green \"begin\" button") -> ()  [unwired: 1 in, 1 out]
    }
    frame #2 {
      # "Allows 5 seconds\n to change it before\n asking again"
      n140 = while {
        tunnel: ["Cooling Temp"] -> w410
        stop <- w417 stop-if-true
        n141 = Number To Decimal String(number="Cooling Temp") -> (decimal integer string=w416:string)  [unwired: 1 in]
        n142 = Concatenate Strings("Is the temperature ", w416, " correct?") -> (w413:string)
        n143 = Two Button Dialog(message=w413) -> (T button?=w417:bool)  [unwired: 2 in]
        n144 = case shown="True" w417 {
          frame False {
            n145 = Wait (ms)(milliseconds to wait=5000) -> ()  [unwired: 1 out]
          }
          frame True {
          }
        }
      }
    }
    frame #3 {
      n146 = call <userlib>:"CameraSetTemp.vi"("error in (no error)"=w421, "Temperature"=w419, "Camera Handle"=w423) -> ("error out"=w420:errorcluster, "Camera Handle"=w422:u32)
      n147 = Two Button Dialog(message="Would you like to home the motors?", 1:"No") -> (T button?=w424:bool)  [unwired: 1 in]
      n148 = while {
        stop <- "begin" stop-if-true
        # "Wait for \nbutton press"
      }
      n149 = while {
        tunnel: w420 -> [w435]
        tunnel: w419 -> [w434]
        tunnel: [w431] -> w427
        tunnel: w422 -> [w430]
        stop <- w433 stop-if-true
        n150 = call <userlib>:"CameraGetTemp.vi"("Camera Handle"=w430, "error in (no error)"=w435) -> ("Temperature"=w432:dbl, "error out"=w431:errorcluster)  [unwired: 1 out]
        "Read Temp" <- w432
        n151 = Equal?(x=w432, y=w434) -> (x = y?=w433:bool)
        n152 = Wait (ms)(milliseconds to wait=1000) -> ()  [unwired: 1 out]
      }
    }
    frame #4 {
      n153 = Bundle("Detector X Start"="Detector X Start", "Detector Y Start"="Detector Y Start", "Grating X Start"="Grating X Start", "Grating Y Start"="Grating Y Start", "Grating Angle Start"="Grating Angle Start", "Aperture X Start"="Aperture X Start", "Polarization Start"="Polarization Start", "Mirror X Start"="Mirror X Start", "Mirror Angle Start"="Mirror Angle Start") -> (w463:T8)  [unwired: 1 in]
      n154 = Bundle("Detector X End"="Detector X End", "Detector Y End"="Detector Y End", "Grating X End"="Grating X End", "Grating Y End"="Grating Y End", "Grating Angle End"="Grating Angle End", "Aperture X End"="Aperture X End", "Polarization End"="Polarization End", "Mirror X End"="Mirror X End", "Mirror Angle End"="Mirror Angle End") -> (w443:T9)  [unwired: 1 in]
      n155 = Bundle("Detector X#Steps"="Detector X#Steps", "Detector Y#Steps"="Detector Y#Steps", "Grating X#Steps"="Grating X#Steps", "Grating Y#Steps"="Grating Y#Steps", "Grating Angle#Steps"="Grating Angle#Steps", "Aperture X#Steps"="Aperture X#Steps", "Polarization #Steps"="Polarization #Steps", "Mirror X #Steps"="Mirror X #Steps", "Mirror Angle #Steps"="Mirror Angle #Steps") -> (w436:T10)  [unwired: 1 in]
      n156 = Bundle("ADC Speed (kHz)"="ADC Speed (kHz)", "Throwaway Frames"="Throwaway Frames", "# Frames"="# Frames", "Exposure"="Exposure", "Cooling Temp"=w441) -> (w440:T11)  [unwired: 1 in]
      n157 = Bundle("X1"="X1", "X2"="X2", "x bin"="x bin", "Y1"="Y1", "Y2"="Y2", "y bin"="y bin") -> (w475:T12)  [unwired: 1 in]
    }
    frame #5 {
      n158 = global read "CamHandle.vi" "Cam Handle"() -> (w508:u32)
      n159 = call <userlib>:"CameraSkips.vi"("Camera Handle"=w508, "Minimum Block Size"=w507, "Number of Minimum blocks"=w506, "error in"=w504, "Type of Skips"=1) -> ("Camera Handle"=w502:u32, "error out"=w503:errorcluster)
      n160 = Two Button Dialog(message="Make sure the high voltage is turned on, then proceed.\nOtherwise, click \"Voltage is off\" to proceed without a stats file.", 1:"Voltage is off") -> (T button?=→"Logging Indicator":bool)  [unwired: 1 in]
      n161 = call "ExSub1strip.vi"("error in (no error)"=w503, "strip 1"=w489, "Camera Handle"=w502) -> ("error out"=w500:errorcluster, "Camera Handle"=w501:u32)
      n162 = call "ExSubSetup.vi"("error in (no error)"=w500, "Camera Handle"=w501) -> ("error out"=w498:errorcluster, "Camera Handle"=w499:u32)
      n163 = call <userlib>:"CameraTrigger.vi"("error in"=w498, "Trigger Edge"=2, "Timing Mode"="Timing Mode", "Camera Handle"=w499) -> ("Camera Handle"=w495:u32)  [unwired: 1 out]
      n164 = call <userlib>:"CameraADCset.vi"("ADC offset"=-1, "Read Out port"=w492, "ADC Gain"=w490, "ADC Speed"=w494, "Camera Handle"=w495) -> ("error out"=→"error out (ADC)":errorcluster)  [unwired: 1 in, 1 out]
    }
  }
  n165 = while {
    tunnel: 1000 -> [w509]
    stop <- w510 stop-if-true
    n166 = event shown="[0] Timeout" {
      selector: _ -> [_]
      dyn-events: _ -> [_]
      timeout: w509 -> [_]
      tunnel: [FALSE] -> w510
      event Timeout {
        # "When setup, use\nAIN2 for diode 3"
        n167 = event-data() -> ()  [unwired: 1 in, 1 out]
        n168 = local read "Logging Indicator"() -> (w518:bool)
        n169 = case shown="False" w518 {
          frame False {
          }
          frame True {
            w525 = u16 0 items=["Voltage and Current", "Voltage Only", "Current Only"] ("Measure")
            n170 = call "ReadVoltage.vi"("Measure"=w525, "Address"=i16 3) -> ("Current"=w523:dbl, "Voltage"=→"Source Voltage":dbl)
            n171 = Multiply(x=w523, y=1000.0) -> (x*y=→"Current (mA)":dbl)
          }
        }
        n172 = call "U3 eAIN Read Diode Voltage.vi"("Channel-P"=0) -> ("Output Voltage"=w514:dbl)  [unwired: 9 in, 1 out]
        n173 = call "U3 eAIN Read Diode Voltage.vi"("Channel-P"=1) -> ("Output Voltage"=w512:dbl)  [unwired: 9 in, 1 out]
        n174 = Number To Fractional String(number=w514, precision (6)=i16 2) -> (F-format string=→"Diode 2":string)  [unwired: 2 in]
        n175 = Number To Fractional String(number=w512, precision (6)=i16 2) -> (F-format string=→"Diode 1":string)  [unwired: 2 in]
      }
    }
  }
  n176 = Cluster To Array(cluster=w5) -> (array=w10:i32[])
  n177 = Not(x=w95) -> (.not. x?=→"Experiment \nStarted":bool)
  n178 = Multiply Array Elements(1:w10) -> (0:w9:i32)
  n179 = while {
    tunnel: 3000 -> [w538]
    shift-right: [w535] -> w14
    shift-left: errorcluster {"status"=FALSE, "code"=0, "source"=""} ("error out") -> [w536]
    tunnel: w9 -> [w532]
    stop <- w537 stop-if-true
    n180 = event shown="[0] Timeout" {
      selector: _ -> [_]
      dyn-events: _ -> [_]
      timeout: w538 -> [_]
      tunnel: [FALSE] -> w537
      tunnel: [w541] -> w535
      tunnel: w536 -> [w540]
      event Timeout {
        n181 = event-data() -> ()  [unwired: 1 in, 1 out]
        n182 = local read "Logging Indicator"() -> (w542:bool)
        n183 = local read "Axis Positions"() -> (w543:T1)
        n184 = case shown="True" w542 {
          tunnel: w543 -> [_ w565]
          tunnel: [w545 w572] -> w541
          tunnel: w540 -> [w545 w571]
          tunnel: "File Path for Data Log" -> [_ w568]
          frame False {
          }
          frame True {
            w552 = "\t"
            n185 = Unbundle By Name(w565) -> ("Source Anode Rotation (P)"=w573:dbl, "Polarization Angle (P)"=w577:dbl)
            n186 = Open/Create/Replace File(file path (use dialog)=w568, error in=w571, operation (0:open)=T7."open or create") -> (refnum out=w583:refnum<file>, error out=w584:errorcluster)  [unwired: 4 out]
            n187 = Unbundle By Name(w565) -> ("Aperture Translation (P)"=w562:dbl, "Grating Translation (P)"=w561:dbl, "Source Mirror Rotation (P)"=w563:dbl, "Grating Rotation (P)"=w557:dbl, "Camera Translation (P)"=w556:dbl, "Camera Vertical (P)"=w555:dbl, "Grating Vertical (P)"=w553:dbl, "Detector Mirror Rotation (P)"=w554:dbl)
            n188 = Set File Position(refnum=w583, from (0:start)=enum16{"start", "end", "current"}."end", error in=w584) -> (refnum out=w576:refnum<file>, error out=w570:errorcluster)  [unwired: 1 out]
            n189 = local read "Source Voltage"() -> (w566:dbl)
            n190 = local read "Current (mA)"() -> (w567:dbl)
            n191 = local read "Source Mirror Position (mm)"() -> (w569:dbl)
            n192 = local read "Diode 1"() -> (w558:string)
            n193 = local read "Diode 2"() -> (w551:string)
            n194 = local read "Current File"() -> (w549:string)
            n195 = Get Date/Time In Seconds() -> (seconds since 1Jan1904=w581:timestamp)
            n196 = Format Date/Time String(time format string (%c)="%Y-%m-%d %H:%M:%S", seconds (now)=w581) -> (date/time string=w579:string)  [unwired: 1 out]
            n197 = Format Into String(format string=" %7.1f %7.4f %+7.2f %7d %7.2f %7.2f %7.3f %7.3f %7.3f %7.3f %7.3f %7.3f %7.3f", initial string=w579, w566, w567, w577, w573, w569, w563, w562, w561, w557, w556, w555, w554, w553) -> (resulting string=w560:string)  [unwired: 1 in, 1 out]
            n198 = Concatenate Strings("\"", w549, "\"") -> (w546:string)
            n199 = Concatenate Strings(w560, w552, w558, w552, w551, w552, w546, "\r") -> (w559:string)
            n200 = Write to Text File(file (use dialog)=w576, text=w559, error in=w570) -> (refnum out=w575:refnum<file>, error out=w574:errorcluster)  [unwired: 2 out]
            n201 = Close File(refnum=w575, error in=w574) -> (error out=w572:errorcluster)  [unwired: 1 out]
          }
        }
      }
    }
    n202 = local read "Throwaway Frames"() -> (w530:i32)
    n203 = local read "# Frames"() -> (w531:i32)
    n204 = local read "Current Set"() -> (w533:dbl)
    n205 = local read "Current Frame"() -> (w534:dbl)
    n206 = Add(x=w531, y=w530) -> (x+y=w529:i32)
    n207 = call "ProgressBar.vi"("Frames/set"=w529, "#Sets"=w532, "Curren Frame"=w534, "Current Set"=w533) -> ("Progress"=→"Progress":u8, 3:→"?":dbl)  [unwired: 6 in]
  }
  n208 = call <vilib>:"Simple Error Handler.vi"("error in (no error)"=w14) -> ()  [unwired: 4 in, 5 out]
  n209 = local write "Initializing"(w95) -> ()
  n210 = Unbundle By Name(w5) -> ("Detector X#Steps"=w104:i32, "Detector Y#Steps"=w103:i32, "Grating X#Steps"=w102:i32, "Grating Y#Steps"=w101:i32, "Grating Angle#Steps"=w100:i32, "Aperture X#Steps"=w99:i32, "Polarization #Steps"=w98:i32, "Mirror X #Steps"=w97:i32, "Mirror Angle #Steps"=w96:i32)
  n211 = call "timeEstimate.vi"("Cluster"=w5, "Exposure"=w33, "Throwaway Frames"=w35, "#Frames"=w34) -> ("Time"=w19:dbl)  [unwired: 7 in]
  n212 = Round Toward +Infinity(x=w19) -> (ceil(x): smallest int >= x=w18:dbl)
  "Estimated time (min)" <- w18
  n213 = while {
    tunnel: 60000 -> [w588]
    shift-right: [w586] -> _
    shift-left: w18 -> [w587]
    stop <- w585 stop-if-true
    n214 = event shown="[0] Timeout" {
      selector: _ -> [_ _]
      dyn-events: _ -> [_ _]
      timeout: w588 -> [_ _]
      tunnel: w587 -> [w590 _]
      tunnel: [w589 _] -> w586
      tunnel: [_ TRUE] -> w585
      event Timeout {
        n215 = event-data() -> ()  [unwired: 1 in, 3 out]
        n216 = Decrement(x=w590) -> (x-1=w589:dbl)
        n217 = local write "Estimated time (min)"(w589) -> ()
      }
      event "Experiment Complete": Value Change {
        n218 = event-data() -> ()  [unwired: 1 in, 6 out]
        n219 = local write "Estimated time (min)"(0) -> ()
      }
    }
  }
  n220 = Unbundle By Name(w43) -> ("X1"=w42:i32, "X2"=w41:i32, "Y1"=w40:i32, "Y2"=w39:i32)  [unwired: 2 out]
  n221 = Unbundle By Name(w5) -> ("Detector X#Steps"=w78:i32, "Detector Y#Steps"=w77:i32, "Grating X#Steps"=w76:i32, "Grating Y#Steps"=w75:i32, "Grating Angle#Steps"=w74:i32, "Aperture X#Steps"=w73:i32, "Polarization #Steps"=w72:i32, "Mirror X #Steps"=w71:i32, "Mirror Angle #Steps"=w70:i32)
  n222 = Unbundle By Name(w50) -> ("Detector X Start"=w69:dbl, "Detector Y Start"=w68:dbl, "Grating X Start"=w67:dbl, "Grating Y Start"=w66:dbl, "Grating Angle Start"=w65:dbl, "Aperture X Start"=w64:dbl, "Polarization Start"=w63:dbl, "Mirror X Start"=w62:dbl, "Mirror Angle Start"=w61:dbl)
  n223 = Unbundle By Name(w31) -> ("Detector X End"=w60:dbl, "Detector Y End"=w59:dbl, "Grating X End"=w58:dbl, "Grating Y End"=w57:dbl, "Grating Angle End"=w56:dbl, "Aperture X End"=w55:dbl, "Polarization End"=w54:dbl, "Mirror X End"=w53:dbl, "Mirror Angle End"=w52:dbl)
  n224 = Number To Decimal String(number=w42) -> (decimal integer string=w48:string)  [unwired: 1 in]
  n225 = Number To Decimal String(number=w41) -> (decimal integer string=w47:string)  [unwired: 1 in]
  n226 = Number To Decimal String(number=w40) -> (decimal integer string=w46:string)  [unwired: 1 in]
  n227 = Number To Decimal String(number=w39) -> (decimal integer string=w44:string)  [unwired: 1 in]
  n228 = call <vilib>:"Space Constant.vi"() -> ("String"=w45:string)
  n229 = Concatenate Strings("ROI: ", w48, w45, w47, w45, w46, w45, w44) -> (w36:string)
  n230 = call "incrementCalc.vi"("End"=w53, "Start"=w62, "#Steps"=w71) -> ("Increment"=w80:dbl)  [unwired: 7 in, 1 out]
  n231 = call "incrementCalc.vi"("End"=w52, "Start"=w61, "#Steps"=w70) -> ("Increment"=w79:dbl)  [unwired: 7 in, 1 out]
  n232 = call "incrementCalc.vi"("End"=w54, "Start"=w63, "#Steps"=w72) -> ("Increment"=w81:dbl)  [unwired: 7 in, 1 out]
  n233 = call "incrementCalc.vi"("End"=w60, "Start"=w69, "#Steps"=w78) -> ("Increment"=w87:dbl)  [unwired: 7 in, 1 out]
  n234 = call "incrementCalc.vi"("End"=w56, "Start"=w65, "#Steps"=w74) -> ("Increment"=w83:dbl)  [unwired: 7 in, 1 out]
  n235 = call "incrementCalc.vi"("End"=w55, "Start"=w64, "#Steps"=w73) -> ("Increment"=w82:dbl)  [unwired: 7 in, 1 out]
  n236 = call "incrementCalc.vi"("End"=w58, "Start"=w67, "#Steps"=w76) -> ("Increment"=w85:dbl)  [unwired: 7 in, 1 out]
  n237 = call "incrementCalc.vi"("End"=w59, "Start"=w68, "#Steps"=w77) -> ("Increment"=w86:dbl)  [unwired: 7 in, 1 out]
  n238 = call "incrementCalc.vi"("End"=w57, "Start"=w66, "#Steps"=w75) -> ("Increment"=w84:dbl)  [unwired: 7 in, 1 out]
  n239 = flat-sequence {
    tunnel: w24 -> [w602]
    tunnel: w17 -> [w594]
    tunnel: [w593] -> w1
    tunnel: w1 -> [w611]
    frame #0 {
      n240 = local read "Axis Positions"() -> (w595:T1)
      n241 = case shown="False" w602 {
        selector: w602 -> [w603 w604]
        tunnel: [w603 w604] -> w593
        frame False {
        }
        frame True {
          n242 = global read "CamHandle.vi" "Cam Handle"() -> (w605:u32)
          n243 = call "ExSetTemperature.vi"("Temperature"=20) -> ()  [unwired: 2 in, 1 out]
          n244 = while {
            tunnel: w605 -> [w610]
            stop <- w609 stop-if-true
            n245 = call <userlib>:"CameraGetTemp.vi"("Camera Handle"=w610) -> ("Temperature"=w608:dbl)  [unwired: 1 in, 2 out]
            n246 = Greater?(x=w608, y=15) -> (0:w609:bool)
            n247 = local write "Read Temp"(w608) -> ()
          }
        }
      }
      n248 = Open/Create/Replace Datalog(5:w595, 11:w594) -> (0:w601:errorcluster, 3:w600:refnum<k1>)  [unwired: 4 in, 1 out]
      n249 = Set Datalog Position(4:w601, 7:w600) -> (0:w598:errorcluster, 3:w599:refnum<k1>)  [unwired: 2 in]
      n250 = Write Datalog(4:w598, 6:w595, 7:w599) -> (0:w597:errorcluster, 3:w596:refnum<k1>)
      n251 = Close File(refnum=w596, error in=w597) -> ()  [unwired: 2 out]
    }
    frame #1 {
      n252 = case shown="False" w611 {
        frame False {
          n253 = Stop(stop? (T)=TRUE) -> ()
        }
        frame True {
          n254 = global read "CamHandle.vi" "Cam Handle"() -> (w615:u32)
          n255 = call <userlib>:"CameraClose.vi"("Camera Handle"=w615) -> ("error out"=w614:errorcluster)  [unwired: 1 in]
          n256 = flat-sequence {
            tunnel: TRUE -> [w622]
            tunnel: w616 -> [_]
            tunnel: ["Camera off"] -> w617
            frame #0 {
              w621 = 0
              n257 = local write "Camera open"(FALSE) -> ()
              n258 = global write "CamHandle.vi" "Cam Handle"(w621) -> ()
              n259 = global write "CamHandle.vi" "X dimension"(w621) -> ()
              n260 = global write "CamHandle.vi" "Y dimension"(w621) -> ()
              "Camera\nClosed" <- w622
            }
          }
          n261 = call <userlib>:"UninitToolkit.vi"("error in"=w614) -> ("error out"=w616:errorcluster)
          "error out (Shutoff)" <- w616
          n262 = One Button Dialog(message=w617) -> (true=w618:bool)  [unwired: 1 in]
          n263 = Stop(stop? (T)=w618) -> ()
        }
      }
    }
  }
  n264 = Bundle("Increment"=w87, "Increment"=w86, "Increment"=w85, "Increment"=w84, "Increment"=w83, "Increment"=w82, "Increment"=w81, "Increment"=w80, "Increment"=w79) -> (w32:T13)  [unwired: 1 in]
  n265 = for {
    N: w104 -> [_]
    tunnel: w103 -> [w648]
    tunnel: w102 -> [w647]
    tunnel: w101 -> [w646]
    tunnel: w100 -> [w645]
    tunnel: w99 -> [w644]
    tunnel: w98 -> [w643]
    tunnel: w97 -> [w642]
    tunnel: w96 -> [w641]
    tunnel: [FALSE] -> w93 mode=indexing
    tunnel: w17 -> [w639]
    tunnel: w91 -> [w637]
    tunnel: w50 -> [w632]
    shift-right: [w631] -> _
    shift-left: errorcluster {"status"=FALSE, "code"=0, "source"=""} ("error constant") -> [w638]
    tunnel: w37 -> [w636]
    tunnel: w36 -> [w635]
    tunnel: w32 -> [w634]
    tunnel: w31 -> [w633]
    tunnel: w30 -> [w630]
    tunnel: w29 -> [w629]
    tunnel: w28 -> [w628]
    tunnel: w22 -> [w627]
    tunnel: w12 -> [w626]
    tunnel: w11 -> [w625]
    tunnel: [w623] -> _ mode=indexing
    tunnel: [w623] -> w4 mode=indexing
    w623 = 100
    n266 = local read "Current Set"() -> (w624:dbl)
    n267 = stacked-sequence {
      tunnel: w648 -> [w672 _]
      tunnel: w647 -> [w671 _]
      tunnel: w646 -> [w670 _]
      tunnel: w645 -> [w669 _]
      tunnel: w644 -> [w668 _]
      tunnel: w643 -> [w667 _]
      tunnel: w642 -> [w666 _]
      tunnel: w641 -> [w665 _]
      tunnel: w639 -> [w664 _]
      tunnel: w638 -> [w663 _]
      tunnel: w637 -> [w662 _]
      tunnel: w636 -> [w661 _]
      tunnel: w635 -> [w660 _]
      tunnel: w634 -> [w659 w1190]
      tunnel: w633 -> [w658 w1198]
      tunnel: w632 -> [w657 w1197]
      tunnel: [w656 _] -> w631
      tunnel: w624 -> [w655 _]
      tunnel: [w654 _] -> _
      tunnel: w630 -> [w653 _]
      tunnel: w629 -> [w652 _]
      tunnel: w628 -> [w651 _]
      tunnel: w627 -> [w650 _]
      tunnel: w626 -> [w649 _]
      tunnel: w625 -> [_ w1194]
      frame #0 {
        n268 = for {
          N: w672 -> [_]
          tunnel: w671 -> [w695]
          tunnel: w670 -> [w694]
          tunnel: w669 -> [w693]
          tunnel: w668 -> [w692]
          tunnel: w667 -> [w691]
          tunnel: w666 -> [w690]
          tunnel: w665 -> [w689]
          tunnel: w664 -> [w688]
          shift-right: [w686] -> w656
          shift-left: w663 -> [w687]
          tunnel: w662 -> [w685]
          tunnel: w661 -> [w684]
          tunnel: w660 -> [w683]
          tunnel: w659 -> [w682]
          tunnel: w658 -> [w681]
          tunnel: w657 -> [w680]
          shift-right: [w678] -> w654
          shift-left: w655 -> [w679]
          tunnel: w653 -> [w677]
          tunnel: w652 -> [w676]
          tunnel: w651 -> [w675]
          tunnel: w650 -> [w674]
          tunnel: w649 -> [w673]
          n269 = stacked-sequence {
            tunnel: w695 -> [w717 _]
            tunnel: w694 -> [w716 _]
            tunnel: w693 -> [w715 _]
            tunnel: w692 -> [w714 _]
            tunnel: w691 -> [w713 _]
            tunnel: w690 -> [w712 _]
            tunnel: w689 -> [w711 _]
            tunnel: w688 -> [w710 _]
            tunnel: w687 -> [w709 _]
            tunnel: [w708 _] -> w686
            tunnel: w685 -> [w707 _]
            tunnel: w684 -> [w706 _]
            tunnel: w683 -> [w705 _]
            tunnel: w682 -> [w704 w1167]
            tunnel: w681 -> [w703 w1174]
            tunnel: w680 -> [w702 w1175]
            tunnel: w679 -> [w701 _]
            tunnel: [w700 _] -> w678
            tunnel: w677 -> [w699 _]
            tunnel: w676 -> [w698 _]
            tunnel: w675 -> [w697 _]
            tunnel: w674 -> [w696 _]
            tunnel: w673 -> [_ w1170]
            frame #0 {
              n270 = for {
                N: w717 -> [_]
                tunnel: w716 -> [w738]
                tunnel: w715 -> [w737]
                tunnel: w714 -> [w736]
                tunnel: w713 -> [w735]
                tunnel: w712 -> [w734]
                tunnel: w711 -> [w733]
                tunnel: w710 -> [w732]
                shift-right: [w730] -> w708
                shift-left: w709 -> [w731]
                tunnel: w707 -> [w729]
                tunnel: w706 -> [w728]
                tunnel: w705 -> [w727]
                tunnel: w704 -> [w726]
                tunnel: w703 -> [w725]
                tunnel: w702 -> [w724]
                shift-right: [w722] -> w700
                shift-left: w701 -> [w723]
                tunnel: w699 -> [w721]
                tunnel: w698 -> [w720]
                tunnel: w697 -> [w719]
                tunnel: w696 -> [w718]
                n271 = stacked-sequence {
                  tunnel: w738 -> [w758 _]
                  tunnel: w737 -> [w757 _]
                  tunnel: w736 -> [w756 _]
                  tunnel: w735 -> [w755 _]
                  tunnel: w734 -> [w754 _]
                  tunnel: w733 -> [w753 _]
                  tunnel: w732 -> [w752 _]
                  tunnel: w731 -> [w751 _]
                  tunnel: [w750 _] -> w730
                  tunnel: w729 -> [w749 _]
                  tunnel: w728 -> [w748 _]
                  tunnel: w727 -> [w747 _]
                  tunnel: w726 -> [w746 w1143]
                  tunnel: w725 -> [w745 w1152]
                  tunnel: w724 -> [w744 w1149]
                  tunnel: w723 -> [w743 _]
                  tunnel: [w742 _] -> w722
                  tunnel: w721 -> [w741 _]
                  tunnel: w720 -> [w740 _]
                  tunnel: w719 -> [w739 _]
                  tunnel: w718 -> [_ w1146]
                  frame #0 {
                    n272 = for {
                      N: w758 -> [_]
                      tunnel: w757 -> [w777]
                      tunnel: w756 -> [w776]
                      tunnel: w755 -> [w775]
                      tunnel: w754 -> [w774]
                      tunnel: w753 -> [w773]
                      tunnel: w752 -> [w772]
                      shift-right: [w770] -> w750
                      shift-left: w751 -> [w771]
                      tunnel: w749 -> [w769]
                      tunnel: w748 -> [w768]
                      tunnel: w747 -> [w767]
                      tunnel: w746 -> [w766]
                      tunnel: w745 -> [w765]
                      tunnel: w744 -> [w764]
                      shift-right: [w762] -> w742
                      shift-left: w743 -> [w763]
                      tunnel: w741 -> [w761]
                      tunnel: w740 -> [w760]
                      tunnel: w739 -> [w759]
                      n273 = stacked-sequence {
                        tunnel: w777 -> [w795 _]
                        tunnel: w776 -> [w794 _]
                        tunnel: w775 -> [w793 _]
                        tunnel: w774 -> [w792 _]
                        tunnel: w773 -> [w791 _]
                        tunnel: w772 -> [w790 _]
                        tunnel: w771 -> [w789 _]
                        tunnel: [w788 _] -> w770
                        tunnel: w769 -> [w787 _]
                        tunnel: w768 -> [w786 _]
                        tunnel: w767 -> [w785 _]
                        tunnel: w766 -> [w784 w1119]
                        tunnel: w765 -> [w783 w1126]
                        tunnel: w764 -> [w782 w1127]
                        tunnel: w763 -> [w781 _]
                        tunnel: [w780 _] -> w762
                        tunnel: w761 -> [w779 _]
                        tunnel: w760 -> [w778 _]
                        tunnel: w759 -> [_ w1122]
                        frame #0 {
                          n274 = for {
                            N: w795 -> [_]
                            tunnel: w794 -> [w812]
                            tunnel: w793 -> [w811]
                            tunnel: w792 -> [w810]
                            tunnel: w791 -> [w809]
                            tunnel: w790 -> [w808]
                            shift-right: [w806] -> w788
                            shift-left: w789 -> [w807]
                            tunnel: w787 -> [w805]
                            tunnel: w786 -> [w804]
                            tunnel: w785 -> [w803]
                            tunnel: w784 -> [w802]
                            tunnel: w783 -> [w801]
                            tunnel: w782 -> [w800]
                            shift-right: [w798] -> w780
                            shift-left: w781 -> [w799]
                            tunnel: w779 -> [w797]
                            tunnel: w778 -> [w796]
                            n275 = stacked-sequence {
                              tunnel: w812 -> [w828 _]
                              tunnel: w811 -> [w827 _]
                              tunnel: w810 -> [w826 _]
                              tunnel: w809 -> [w825 _]
                              tunnel: w808 -> [w824 _]
                              tunnel: w807 -> [w823 _]
                              tunnel: [w822 _] -> w806
                              tunnel: w805 -> [w821 _]
                              tunnel: w804 -> [w820 _]
                              tunnel: w803 -> [w819 _]
                              tunnel: w802 -> [w818 w1098]
                              tunnel: w801 -> [w817 w1106]
                              tunnel: w800 -> [w816 w1107]
                              tunnel: w799 -> [w815 _]
                              tunnel: [w814 _] -> w798
                              tunnel: w797 -> [w813 _]
                              tunnel: w796 -> [_ w1101]
                              frame #0 {
                                n276 = for {
                                N: w828 -> [_]
                                tunnel: w827 -> [w843]
                                tunnel: w826 -> [w842]
                                tunnel: w825 -> [w841]
                                tunnel: w824 -> [w840]
                                shift-right: [w838] -> w822
                                shift-left: w823 -> [w839]
                                tunnel: w821 -> [w837]
                                tunnel: w820 -> [w836]
                                tunnel: w819 -> [w835]
                                tunnel: w818 -> [w834]
                                tunnel: w817 -> [w833]
                                tunnel: w816 -> [w832]
                                shift-right: [w830] -> w814
                                shift-left: w815 -> [w831]
                                tunnel: w813 -> [w829]
                                n277 = stacked-sequence {
                                tunnel: w843 -> [w857 _]
                                tunnel: w842 -> [w856 _]
                                tunnel: w841 -> [w855 _]
                                tunnel: w840 -> [w854 _]
                                tunnel: w839 -> [w853 _]
                                tunnel: [w852 _] -> w838
                                tunnel: w837 -> [w851 _]
                                tunnel: w836 -> [w850 _]
                                tunnel: w835 -> [w849 _]
                                tunnel: w834 -> [w848 w1082]
                                tunnel: w833 -> [w847 w1081]
                                tunnel: w832 -> [w846 w1083]
                                tunnel: w831 -> [w845 _]
                                tunnel: [w844 _] -> w830
                                tunnel: w829 -> [_ w1075]
                                frame #0 {
                                n278 = for {
                                N: w857 -> [_]
                                tunnel: w856 -> [w870]
                                tunnel: w855 -> [w869]
                                tunnel: w854 -> [w868]
                                shift-right: [w866] -> w852
                                shift-left: w853 -> [w867]
                                tunnel: w851 -> [w865]
                                tunnel: w850 -> [w864]
                                tunnel: w849 -> [w863]
                                tunnel: w848 -> [w862]
                                tunnel: w847 -> [w861]
                                tunnel: w846 -> [w860]
                                shift-right: [w858] -> w844
                                shift-left: w845 -> [w859]
                                n279 = stacked-sequence {
                                tunnel: w870 -> [w883 _]
                                tunnel: w869 -> [w882 _]
                                tunnel: w868 -> [w881 _]
                                tunnel: w867 -> [w880 _]
                                tunnel: [w879 _] -> w866
                                tunnel: w865 -> [w878 _]
                                tunnel: w864 -> [w877 _]
                                tunnel: w863 -> [w876 _]
                                tunnel: w862 -> [w875 w1046]
                                tunnel: w861 -> [w874 w1052]
                                tunnel: w860 -> [w873 w1051]
                                tunnel: w859 -> [w872 _]
                                tunnel: [w871 _] -> w858
                                frame #0 {
                                n280 = for {
                                N: w883 -> [_]
                                tunnel: w882 -> [w895]
                                tunnel: w881 -> [w894]
                                shift-right: [w893] -> w879
                                shift-left: w880 -> [w892]
                                tunnel: w878 -> [w891]
                                tunnel: w877 -> [w890]
                                tunnel: w876 -> [w889]
                                tunnel: w875 -> [w888]
                                tunnel: w874 -> [w887]
                                tunnel: w873 -> [w886]
                                shift-right: [w884] -> w871
                                shift-left: w872 -> [w885]
                                n281 = stacked-sequence {
                                tunnel: w895 -> [w907 w1014]
                                tunnel: w894 -> [w906 _]
                                tunnel: [w905 _] -> w893
                                tunnel: w892 -> [w904 _]
                                tunnel: w891 -> [w903 _]
                                tunnel: w890 -> [w902 _]
                                tunnel: w889 -> [w901 _]
                                tunnel: w888 -> [w900 w1017]
                                tunnel: w887 -> [w899 w1021]
                                tunnel: w886 -> [w898 w1022]
                                tunnel: w885 -> [w897 _]
                                tunnel: [w896 _] -> w884
                                tunnel: [_ w1014] -> _
                                frame #0 {
                                n282 = for {
                                N: w907 -> [_]
                                shift-right: [w921] -> w905
                                shift-left: w904 -> [w920]
                                tunnel: w906 -> [w922]
                                tunnel: w903 -> [w910]
                                tunnel: w902 -> [w918]
                                tunnel: w901 -> [w917]
                                tunnel: w900 -> [w914]
                                tunnel: w899 -> [w916]
                                tunnel: w898 -> [w915]
                                shift-right: [w912] -> w896
                                shift-left: w897 -> [w913]
                                # "Data and Mirror Angle loop"
                                n283 = call "Check File Path.vi"("Extension"=".tif", "Path to Check"=w910) -> ("Valid Path"=w911:path)  [unwired: 6 in, 3 out]
                                n284 = Path To String(path=w911) -> (string=w909:string)
                                "Current File" <- w909
                                n285 = call "filename.vi"("String"=w909) -> ("Path"=w908:path)  [unwired: 10 in]
                                n286 = stacked-sequence {
                                tunnel: w922 -> [w933 _ _]
                                tunnel: [w927 _ _] -> w921
                                tunnel: w920 -> [w925 w942 _]
                                tunnel: w911 -> [_ w953 _]
                                tunnel: w918 -> [_ w951 _]
                                tunnel: w917 -> [_ w946 _]
                                tunnel: w916 -> [_ _ w990]
                                tunnel: w915 -> [_ _ w983]
                                tunnel: w914 -> [_ _ w985]
                                tunnel: w913 -> [_ w940 _]
                                tunnel: [_ w939 _] -> w912
                                tunnel: w908 -> [_ w936 _]
                                frame #0 {
                                # "Record motor positions\n\nThis is NOT the header file"
                                # "Make this record currPos"
                                n287 = local read "Axis Positions"() -> (w924:T1)
                                n288 = local write "Boolean"(TRUE) -> ()
                                n289 = Open/Create/Replace Datalog(5:w924, 8:w925, 10:T7."open or create" ("operation (0:open)"), 11:w933) -> (0:w935:errorcluster, 3:w934:refnum<k1>)  [unwired: 2 in, 1 out]
                                n290 = Set Datalog Position(4:w935, 5:enum16{"start", "end", "current"}."end" ("from (0:start)"), 7:w934) -> (0:w930:errorcluster, 3:w931:refnum<k1>)  [unwired: 1 in]
                                n291 = Write Datalog(4:w930, 6:w924, 7:w931) -> (0:w929:errorcluster, 3:w928:refnum<k1>)
                                n292 = Close File(refnum=w928, error in=w929) -> (error out=w927:errorcluster)  [unwired: 1 out]
                                }
                                frame #1 {
                                # "This loop counts and displays the frame #"
                                # "Take Data\nand write header"
                                n293 = local read "Axis Positions"() -> (w941:T1)
                                n294 = Unbundle By Name(w941) -> ("Source Anode Rotation (P)"=w968:dbl, "Aperture Translation (P)"=w964:dbl, "Grating Translation (P)"=w961:dbl, "Grating Vertical (P)"=w962:dbl, "Grating Rotation (P)"=w963:dbl, "Polarization Angle (P)"=w965:dbl, "Source Mirror Translation (P)"=w967:dbl, "Source Mirror Rotation (P)"=w966:dbl, "Camera Translation (P)"=w959:dbl, "Camera Vertical (P)"=w960:dbl)  [unwired: 1 out]
                                n295 = Increment(x=w940) -> (x+1=w939:dbl)
                                n296 = local write "Current Set"(w939) -> ()
                                n297 = Get Date/Time String(want seconds? (F)=TRUE) -> (date string=w957:string, time string=w956:string)  [unwired: 2 in]
                                n298 = Path To String(path=w953) -> (string=w952:string)
                                n299 = control-ref of="Experiment \nStarted"() -> (w969:refnum<vi>)
                                n300 = Unbundle By Name(w951) -> ("ADC Speed (kHz)"=w945:i32, "Throwaway Frames"=w948:i32, "# Frames"=w947:i32, "Exposure"=w949:i32, "Cooling Temp"=w943:dbl)
                                n301 = Add(x=w948, y=w947) -> (x+y=w944:i32)
                                n302 = call "TakeData.vi"("Boolean in"=w969, "File Path"=w952, "Exposure"=w949, "Total Frames"=w944, "error in"=w942) -> ("Counter Reset"=w950:i32, "Start Time"=w970:dbl, "End Time"=w971:dbl, "Stop count"=w938:bool, "Start time sec"=w955:dbl, "End Time sec"=w954:dbl, "error out"=w972:errorcluster)  [unwired: 3 in, 1 out]
                                n303 = Not(x=w938) -> (.not. x?=→"Boolean":bool)
                                n304 = call "StoreHeaderMotorInfo.vi"("Temperature"=w943, "StartTime"=w970, "MirrorTrans"=w967, "ROI/Binning String"=w946, "Anode"=w968, "Throwaway Frames"=w948, "MirrorAngle"=w966, "error in (no error)"=w972, "Image Path"=w936, "Number of Images"=w947, "CameraX"=w959, "ADC speed (kHz)"=w945, "Exposure"=w949, "Polarization"=w965, "StartSec"=w955, "EndTime"=w971, "Date String"=w957, "EndSec"=w954, "Aperture"=w964, "GratingAngle"=w963, "GratingY"=w962, "GratingX"=w961, "Time String"=w956, "CameraY"=w960) -> ()  [unwired: 4 in]
                                n305 = while {
                                tunnel: w948 -> [w978]
                                tunnel: w944 -> [w976]
                                stop <- w974 continue-if-true
                                n306 = global read "NumericIndicator.vi" "Iteration"() -> (w979:dbl)
                                n307 = Less?(x=w979, y=w976) -> (x < y?=w975:bool)
                                n308 = local read "Boolean"() -> (w973:bool)
                                n309 = Subtract(x=w979, y=w978) -> (x-y=→"Current Frame":dbl)
                                n310 = And(x=w975, y=w973) -> (x .and. y?=w974:bool)
                                }
                                n311 = local write "Current Frame"(w950) -> ()
                                }
                                frame #2 {
                                # "Move inner motor, mirror angle"
                                n312 = Unbundle By Name(w990) -> ("Mirror Angle End"=w980:dbl)
                                n313 = Unbundle By Name(w983) -> ("Mirror Angle Start"=w981:dbl)
                                n314 = local read "Axis Positions"() -> (w984:T1)
                                n315 = Unbundle By Name(w984) -> ("Source Mirror Rotation (P)"=w988:dbl)
                                n316 = Equal?(x=w980, y=w981) -> (x = y?=w982:bool)
                                n317 = Equal?(x=w988, y=w980) -> (x = y?=w989:bool)
                                n318 = case shown="False" w982 {
                                tunnel: w989 -> [w996 _]
                                tunnel: w988 -> [w995 w1005]
                                tunnel: [w994 w1005] -> w987
                                tunnel: w985 -> [w993 _]
                                tunnel: w981 -> [w992 _]
                                frame False {
                                n319 = case shown="False" w996 {
                                tunnel: w995 -> [w1001 w1004]
                                tunnel: [w997 w1003] -> w994
                                tunnel: w993 -> [w1000 _]
                                tunnel: w992 -> [_ w1002]
                                frame False {
                                # "move to next\npoint"
                                n320 = Unbundle(w1000) -> ("Increment"=w999:dbl)  [unwired: 8 out]
                                n321 = Add(x=w1001, y=w999) -> (x+y=w998:dbl)
                                n322 = call "SourceMirrorAngle.vi"("EndPos"=w998, "CurrPos"=w1001) -> ("Curr Pos"=w997:dbl)  [unwired: 9 in]
                                }
                                frame True {
                                # "loop ended, move\nback to start"
                                n323 = call "SourceMirrorAngle.vi"("EndPos"=w1002, "CurrPos"=w1004) -> ("Curr Pos"=w1003:dbl)  [unwired: 9 in]
                                }
                                }
                                n324 = Wait (ms)(milliseconds to wait=15000) -> ()  [unwired: 1 out]
                                }
                                frame True {
                                }
                                }
                                n325 = Bundle By Name(cluster=w984, "Source Mirror Rotation (P)"=w987) -> (w986:T1)
                                n326 = local write "Axis Positions"(w986) -> ()
                                }
                                }
                                }
                                }
                                frame #1 {
                                # "Move Mirror Trans Motor"
                                n327 = local read "Axis Positions"() -> (w1018:T1)
                                n328 = Unbundle By Name(w1018) -> ("Source Mirror Translation (P)"=w1019:dbl)
                                n329 = Unbundle By Name(w1021) -> ("Mirror X End"=w1012:dbl)
                                n330 = Unbundle By Name(w1022) -> ("Mirror X Start"=w1013:dbl)
                                n331 = Equal?(x=w1012, y=w1019) -> (x = y?=w1020:bool)
                                n332 = Equal?(x=w1013, y=w1012) -> (x = y?=w1011:bool)
                                n333 = case shown="False" w1011 {
                                tunnel: w1020 -> [w1030 _]
                                tunnel: w1019 -> [w1029 w1041]
                                tunnel: w1018 -> [w1028 w1042]
                                tunnel: w1017 -> [w1027 _]
                                tunnel: [w1026 w1042] -> w1016
                                tunnel: [w1025 w1041] -> w1007
                                tunnel: w1013 -> [w1024 _]
                                frame False {
                                n334 = case shown="True" w1030 {
                                tunnel: w1024 -> [_ w1040]
                                tunnel: w1029 -> [w1034 w1039]
                                tunnel: [w1032 w1038] -> w1026
                                tunnel: w1028 -> [w1032 w1038]
                                tunnel: w1027 -> [w1036 _]
                                tunnel: [w1031 w1037] -> w1025
                                frame False {
                                # "Moves forward *increment*"
                                n335 = Unbundle(w1036) -> ("Increment"=w1035:dbl)  [unwired: 8 out]
                                n336 = Add(x=w1035, y=w1034) -> (x+y=w1033:dbl)
                                n337 = call "SourceMirrorTrans.vi"("EndPos"=w1033, "CurrPos"=w1034) -> ("Curr Pos"=w1031:dbl)  [unwired: 9 in]
                                }
                                frame True {
                                # "Moves Back to Start"
                                n338 = call "SourceMirrorTrans.vi"("EndPos"=w1040, "CurrPos"=w1039) -> ("Curr Pos"=w1037:dbl)  [unwired: 9 in]
                                }
                                }
                                n339 = Wait (ms)(milliseconds to wait=15000) -> ()  [unwired: 1 out]
                                }
                                frame True {
                                }
                                }
                                n340 = Subtract(x=3.7594, y=w1007) -> (x-y=w1006:dbl)
                                n341 = Bundle By Name(cluster=w1016, "Source Mirror Translation (P)"=w1007) -> (w1015:T1)
                                n342 = Multiply(x=25.4, y=w1006) -> (x*y=w1010:dbl)
                                n343 = local write "Axis Positions"(w1015) -> ()
                                n344 = local write "Source Mirror Position (mm)"(w1010) -> ()
                                }
                                }
                                }
                                }
                                frame #1 {
                                # "Move Polarization Motor"
                                n345 = local read "Axis Positions"() -> (w1053:T1)
                                n346 = Unbundle By Name(w1053) -> ("Polarization Angle (P)"=w1050:dbl)
                                n347 = Unbundle By Name(w1051) -> ("Polarization Start"=w1044:dbl)
                                n348 = Unbundle By Name(w1052) -> ("Polarization End"=w1045:dbl)
                                n349 = Equal?(x=w1050, y=w1045) -> (x = y?=w1054:bool)
                                n350 = Equal?(x=w1045, y=w1044) -> (x = y?=w1043:bool)
                                n351 = case shown="False" w1043 {
                                tunnel: w1054 -> [w1060 _]
                                tunnel: w1044 -> [w1059 _]
                                tunnel: w1050 -> [w1058 w1069]
                                tunnel: [w1057 w1069] -> w1048
                                tunnel: w1046 -> [w1056 _]
                                frame False {
                                n352 = case shown="True" w1060 {
                                tunnel: w1059 -> [_ w1068]
                                tunnel: w1058 -> [w1065 w1067]
                                tunnel: [w1061 w1066] -> w1057
                                tunnel: w1056 -> [w1064 _]
                                frame False {
                                # "Increment"
                                n353 = Unbundle(w1064) -> ("Increment"=w1063:dbl)  [unwired: 8 out]
                                n354 = Add(x=w1065, y=w1063) -> (x+y=w1062:dbl)
                                n355 = call "RotatePolarization.vi"("End Pos"=w1062, "curr pos"=w1065) -> ("Pos out"=w1061:dbl)  [unwired: 9 in]
                                }
                                frame True {
                                # "Return to start"
                                n356 = call "RotatePolarization.vi"("End Pos"=w1068, "curr pos"=w1067) -> ("Pos out"=w1066:dbl)  [unwired: 9 in]
                                }
                                }
                                n357 = Wait (ms)(milliseconds to wait=15000) -> ()  [unwired: 1 out]
                                }
                                frame True {
                                }
                                }
                                n358 = local read "Axis Positions"() -> (w1049:T1)
                                n359 = Bundle By Name(cluster=w1049, "Polarization Angle (P)"=w1048) -> (w1047:T1)
                                n360 = local write "Axis Positions"(w1047) -> ()
                                }
                                }
                                }
                                }
                                frame #1 {
                                # "Move Aperture Motor"
                                n361 = Unbundle By Name(w1083) -> ("Aperture X Start"=w1076:dbl)
                                n362 = local read "Axis Positions"() -> (w1080:T1)
                                n363 = Unbundle By Name(w1081) -> ("Aperture X End"=w1079:dbl)
                                n364 = Unbundle(w1075) -> ("Axis Prefix"=w1074:string, w1073:i32)  [unwired: 4 out]
                                n365 = Unbundle By Name(w1080) -> ("Aperture Translation (P)"=w1077:dbl)
                                n366 = Equal?(x=w1079, y=w1077) -> (x = y?=w1078:bool)
                                n367 = case shown="False" w1078 {
                                tunnel: w1082 -> [w1089 _]
                                tunnel: w1077 -> [w1086 w1093]
                                tunnel: w1076 -> [_ w1090]
                                tunnel: w1074 -> [w1087 w1092]
                                tunnel: w1073 -> [w1088 w1091]
                                tunnel: [w1084 w1090] -> w1070
                                frame False {
                                n368 = Unbundle(w1089) -> ("Increment"=w1085:dbl)  [unwired: 8 out]
                                n369 = Add(x=w1085, y=w1086) -> (x+y=w1084:dbl)
                                n370 = call "MoveTo.vi"("Curr Pos"=w1086, "Desired Pos"=w1084, "Axis Name"=w1087, "Steps/unit"=w1088) -> ()  [unwired: 7 in, 1 out]
                                }
                                frame True {
                                n371 = call "MoveTo.vi"("Curr Pos"=w1093, "Desired Pos"=w1090, "Axis Name"=w1092, "Steps/unit"=w1091) -> ()  [unwired: 7 in, 1 out]
                                }
                                }
                                n372 = local read "Axis Positions"() -> (w1072:T1)
                                n373 = Bundle By Name(cluster=w1072, "Aperture Translation (P)"=w1070) -> (w1071:T1)
                                n374 = local write "Axis Positions"(w1071) -> ()
                                }
                                }
                                }
                              }
                              frame #1 {
                                n375 = Unbundle By Name(w1107) -> ("Grating Angle Start"=w1103:dbl)
                                n376 = local read "Axis Positions"() -> (w1095:T1)
                                n377 = Unbundle By Name(w1106) -> ("Grating Angle End"=w1105:dbl)
                                n378 = Unbundle By Name(w1095) -> ("Grating Rotation (P)"=w1102:dbl)
                                n379 = Equal?(x=w1105, y=w1102) -> (x = y?=w1104:bool)
                                n380 = Unbundle(w1101) -> ("Axis Prefix"=w1100:string, w1099:i32)  [unwired: 4 out]
                                n381 = Unbundle(w1098) -> ("Increment"=w1097:dbl)  [unwired: 8 out]
                                n382 = case shown="True" w1104 {
                                tunnel: w1103 -> [_ w1112]
                                tunnel: w1102 -> [w1109 w1115]
                                tunnel: w1100 -> [w1111 w1114]
                                tunnel: w1099 -> [w1110 w1113]
                                tunnel: w1097 -> [w1108 _]
                                tunnel: [w1108 w1112] -> w1094
                                frame False {
                                n383 = call "MoveTo.vi"("Curr Pos"=w1109, "Desired Pos"=w1108, "Axis Name"=w1111, "Steps/unit"=w1110) -> ()  [unwired: 7 in, 1 out]
                                }
                                frame True {
                                n384 = call "MoveTo.vi"("Curr Pos"=w1115, "Desired Pos"=w1112, "Axis Name"=w1114, "Steps/unit"=w1113) -> ()  [unwired: 7 in, 1 out]
                                }
                                }
                                n385 = Bundle By Name(cluster=w1095, "Grating Rotation (P)"=w1094) -> (w1096:T1)
                                n386 = local write "Axis Positions"(w1096) -> ()
                              }
                            }
                          }
                        }
                        frame #1 {
                          # "Move Grating Y"
                          n387 = Unbundle By Name(w1127) -> ("Grating Y Start"=w1124:dbl)
                          n388 = local read "Axis Positions"() -> (w1117:T1)
                          n389 = Unbundle(w1122) -> ("Axis Prefix"=w1121:string, w1120:i32)  [unwired: 4 out]
                          n390 = Unbundle By Name(w1117) -> ("Grating Vertical (P)"=w1123:dbl)
                          n391 = Unbundle By Name(w1126) -> ("Grating Y End"=w1125:dbl)
                          n392 = Equal?(x=w1125, y=w1123) -> (x = y?=w1128:bool)
                          n393 = case shown="True" w1128 {
                            tunnel: w1124 -> [_ w1135]
                            tunnel: w1123 -> [w1131 w1138]
                            tunnel: w1121 -> [w1133 w1137]
                            tunnel: w1120 -> [w1134 w1136]
                            tunnel: w1119 -> [w1132 _]
                            tunnel: [w1129 w1135] -> w1116
                            frame False {
                              n394 = Unbundle(w1132) -> ("Increment"=w1130:dbl)  [unwired: 8 out]
                              n395 = Add(x=w1130, y=w1131) -> (x+y=w1129:dbl)
                              n396 = call "MoveTo.vi"("Curr Pos"=w1131, "Desired Pos"=w1129, "Axis Name"=w1133, "Steps/unit"=w1134) -> ()  [unwired: 7 in, 1 out]
                            }
                            frame True {
                              n397 = call "MoveTo.vi"("Curr Pos"=w1138, "Desired Pos"=w1135, "Axis Name"=w1137, "Steps/unit"=w1136) -> ()  [unwired: 7 in, 1 out]
                            }
                          }
                          n398 = Bundle By Name(cluster=w1117, "Grating Vertical (P)"=w1116) -> (w1118:T1)
                          n399 = local write "Axis Positions"(w1118) -> ()
                        }
                      }
                    }
                  }
                  frame #1 {
                    # "Move grating X"
                    n400 = local read "Axis Positions"() -> (w1153:T1)
                    n401 = Unbundle By Name(w1149) -> ("Grating X Start"=w1148:dbl)
                    n402 = Unbundle(w1146) -> ("Axis Prefix"=w1145:string, w1144:i32)  [unwired: 4 out]
                    n403 = Unbundle By Name(w1152) -> ("Grating X End"=w1151:dbl)
                    n404 = Unbundle By Name(w1153) -> ("Grating Translation (P)"=w1147:dbl)
                    n405 = Equal?(x=w1151, y=w1147) -> (x = y?=w1150:bool)
                    n406 = local read "Axis Positions"() -> (w1141:T1)
                    n407 = Unbundle(w1143) -> ("Increment"=w1142:dbl)  [unwired: 8 out]
                    n408 = case shown="True" w1150 {
                      tunnel: w1148 -> [_ w1159]
                      tunnel: w1147 -> [w1155 w1162]
                      tunnel: w1145 -> [w1157 w1161]
                      tunnel: w1144 -> [w1158 w1160]
                      tunnel: w1142 -> [w1156 _]
                      tunnel: [w1154 w1159] -> w1139
                      frame False {
                        n409 = Add(x=w1156, y=w1155) -> (x+y=w1154:dbl)
                        n410 = call "MoveTo.vi"("Curr Pos"=w1155, "Desired Pos"=w1154, "Axis Name"=w1157, "Steps/unit"=w1158) -> ()  [unwired: 7 in, 1 out]
                      }
                      frame True {
                        n411 = call "MoveTo.vi"("Curr Pos"=w1162, "Desired Pos"=w1159, "Axis Name"=w1161, "Steps/unit"=w1160) -> ()  [unwired: 7 in, 1 out]
                      }
                    }
                    n412 = Bundle By Name(cluster=w1141, "Grating Translation (P)"=w1139) -> (w1140:T1)
                    n413 = local write "Axis Positions"(w1140) -> ()
                  }
                }
              }
            }
            frame #1 {
              # "Detector Y move"
              n414 = Unbundle By Name(w1175) -> ("Detector Y Start"=w1172:dbl)
              n415 = local read "Axis Positions"() -> (w1165:T1)
              n416 = Unbundle By Name(w1165) -> ("Camera Vertical (P)"=w1171:dbl)
              n417 = Unbundle By Name(w1174) -> ("Detector Y End"=w1173:dbl)
              n418 = Unbundle(w1170) -> ("Axis Prefix"=w1169:string, w1168:i32)  [unwired: 4 out]
              n419 = Equal?(x=w1173, y=w1171) -> (x = y?=w1176:bool)
              n420 = Unbundle(w1167) -> ("Increment"=w1166:dbl)  [unwired: 8 out]
              n421 = case shown="True" w1176 {
                tunnel: w1172 -> [_ w1182]
                tunnel: w1171 -> [w1178 w1185]
                tunnel: w1169 -> [w1181 w1184]
                tunnel: w1168 -> [w1180 w1183]
                tunnel: w1166 -> [w1179 _]
                tunnel: [w1177 w1182] -> w1164
                frame False {
                  n422 = Add(x=w1179, y=w1178) -> (x+y=w1177:dbl)
                  n423 = call "MoveTo.vi"("Curr Pos"=w1178, "Desired Pos"=w1177, "Axis Name"=w1181, "Steps/unit"=w1180) -> ()  [unwired: 7 in, 1 out]
                }
                frame True {
                  n424 = call "MoveTo.vi"("Curr Pos"=w1185, "Desired Pos"=w1182, "Axis Name"=w1184, "Steps/unit"=w1183) -> ()  [unwired: 7 in, 1 out]
                }
              }
              n425 = Bundle By Name(cluster=w1165, "Camera Vertical (P)"=w1164) -> (w1163:T1)
              n426 = local write "Axis Positions"(w1163) -> ()
            }
          }
        }
      }
      frame #1 {
        # "Move Detector X"
        n427 = Unbundle By Name(w1197) -> ("Detector X Start"=w1195:dbl)
        n428 = local read "Axis Positions"() -> (w1188:T1)
        n429 = Unbundle(w1194) -> ("Axis Prefix"=w1193:string, w1192:i32)  [unwired: 4 out]
        n430 = Unbundle By Name(w1198) -> ("Detector X End"=w1196:dbl)
        n431 = Unbundle By Name(w1188) -> ("Camera Translation (P)"=w1191:dbl)
        n432 = Equal?(x=w1196, y=w1191) -> (x = y?=w1199:bool)
        n433 = Unbundle(w1190) -> ("Increment"=w1189:dbl)  [unwired: 8 out]
        n434 = case shown="True" w1199 {
          tunnel: w1195 -> [_ w1205]
          tunnel: w1193 -> [w1201 w1208]
          tunnel: w1192 -> [w1202 w1207]
          tunnel: w1191 -> [w1203 w1206]
          tunnel: w1189 -> [w1204 _]
          tunnel: [w1200 w1205] -> w1186
          frame False {
            n435 = Add(x=w1204, y=w1203) -> (x+y=w1200:dbl)
            n436 = call "MoveTo.vi"("Curr Pos"=w1203, "Desired Pos"=w1200, "Axis Name"=w1201, "Steps/unit"=w1202) -> ()  [unwired: 7 in, 1 out]
          }
          frame True {
            n437 = call "MoveTo.vi"("Curr Pos"=w1206, "Desired Pos"=w1205, "Axis Name"=w1208, "Steps/unit"=w1207) -> ()  [unwired: 7 in, 1 out]
          }
        }
        n438 = Bundle By Name(cluster=w1188, "Camera Translation (P)"=w1186) -> (w1187:T1)
        n439 = local write "Axis Positions"(w1187) -> ()
      }
    }
  }
  n440 = Index Array(array=w93, index=w3) -> (element=w20:bool)
  n441 = Index Array(array=w4, index=w3) -> (element=w2:i32)
  n442 = local write "Logging Indicator"(w20) -> ()
  n443 = Not(x=w20) -> (.not. x?=w25:bool)
  "Experiment Complete" <- w25
  n444 = local write "Experiment \nStarted"(w20) -> ()
  n445 = local write "Progress"(w2) -> ()
  n446 = case shown="True" w25 {
    tunnel: [w1209 w1212] -> w24
    frame False {
      n447 = Two Button Dialog(message="Warm Camera?", 1:"No") -> (T button?=w1209:bool)  [unwired: 1 in]
    }
    frame True {
      n448 = Two Button Dialog(message="Warm Camera?", 1:"No") -> (T button?=w1212:bool)  [unwired: 1 in]
    }
  }
